vi "Display Lab Panel V9.vi"() -> ()   [LabVIEW 2017]
uses:
  Global display 1.vi
  Global display 3.vi
  Global display 2.vi
panel:
  out "network error":bool
  in  "Tab Control 2":T1(tab)
  out "SIG LAB05-2":T2 {"PF" format="%.2f"; "AMPS" format="%.1f"}
  out "SIG LAB05-1":T2 {"PF" format="%.2f"; "AMPS" format="%.1f"}
  out "SIG LAB04-2":T2 {"PF" format="%.2f"; "AMPS" format="%.1f"}
  out "SIG LAB04-1":T2 {"PF" format="%.2f"; "AMPS" format="%.1f"}
  out "SIG LAB03-2":T2 {"PF" format="%.2f"; "AMPS" format="%.1f"}
  out "SIG LAB03-1":T2 {"PF" format="%.2f"; "AMPS" format="%.1f"}
  out "SIG LAB02-2":T2 {"PF" format="%.2f"; "AMPS" format="%.1f"}
  in  "RUN LAB01-1":bool
  in  "O/I  LAB05-1":bool
  in  "O/I  LAB05-2":bool
  in  "O/I  LAB04-1":bool
  in  "O/I  LAB04-2":bool
  in  "O/I  LAB02-1":bool
  in  "O/I  LAB02-2":bool
  in  "O/I  LAB01-2":bool
  in  "O/I  LAB01-1":bool
  in  "O/I  LAB03-1":bool
  in  "RUN LAB05-2":bool
  in  "RUN LAB05-1":bool
  in  "RUN LAB04-2":bool
  in  "RUN LAB04-1":bool
  in  "RUN LAB03-2":bool
  in  "RUN LAB03-1":bool
  in  "RUN LAB02-2":bool
  in  "RUN LAB02-1":bool
  in  "RUN LAB01-2":bool
  in  "SELECT LAB05-2":T3(radio)
  in  "SELECT LAB05-1":T3(radio)
  in  "SELECT LAB04-2":T3(radio)
  in  "SELECT LAB04-1":T3(radio)
  in  "SELECT LAB03-2":T3(radio)
  in  "SELECT LAB03-1":T3(radio)
  in  "SELECT LAB02-2":T3(radio)
  in  "SELECT LAB02-1":T3(radio)
  in  "SELECT LAB01-2":T3(radio)
  in  "SELECT LAB01-1":T3(radio)
  in  "O/I  LAB03-2":bool
  out "SIG LAB01-1":T2 {"PF" format="%.2f"; "AMPS" format="%.1f"}
  out "SIG LAB01-2":T2 {"PF" format="%.2f"; "AMPS" format="%.1f"}
  out "SIG LAB02-1":T2 {"PF" format="%.2f"; "AMPS" format="%.1f"}
  out "DISP LAB05-2":T4 {"MINS" format="%.2g"}
  out "DISP LAB05-1":T4 {"MINS" format="%.2g"}
  out "DISP LAB04-2":T4 {"MINS" format="%.2g"}
  out "DISP LAB04-1":T4 {"MINS" format="%.2g"}
  out "DISP LAB03-2":T4 {"MINS" format="%.2g"}
  out "DISP LAB03-1":T4 {"MINS" format="%.2g"}
  in  "SET LAB05-2":T5={"NAME"="", "DESCRIPTION"="", "CYCLES"=5.0, "T-RISE mins"=0.0, "T-RISE deg C"=0.0} {"CYCLES" min=5.0 step=1.0}
  in  "SET LAB05-1":T5={"NAME"="", "DESCRIPTION"="", "CYCLES"=5.0, "T-RISE mins"=0.0, "T-RISE deg C"=0.0} {"CYCLES" min=5.0 step=1.0}
  in  "SET LAB04-2":T5={"NAME"="", "DESCRIPTION"="", "CYCLES"=5.0, "T-RISE mins"=0.0, "T-RISE deg C"=0.0} {"CYCLES" min=5.0 step=1.0}
  in  "SET LAB04-1":T5={"NAME"="", "DESCRIPTION"="", "CYCLES"=5.0, "T-RISE mins"=0.0, "T-RISE deg C"=0.0} {"CYCLES" min=5.0 step=1.0}
  in  "SET LAB03-2":T5={"NAME"="", "DESCRIPTION"="", "CYCLES"=5.0, "T-RISE mins"=0.0, "T-RISE deg C"=0.0} {"CYCLES" min=5.0 step=1.0}
  in  "SET LAB03-1":T5={"NAME"="", "DESCRIPTION"="", "CYCLES"=5.0, "T-RISE mins"=0.0, "T-RISE deg C"=0.0} {"CYCLES" min=5.0 step=1.0}
  out "DISP LAB02-2":T4 {"MINS" format="%.2g"}
  out "DISP LAB02-1":T4 {"MINS" format="%.2g"}
  in  "SET LAB02-2":T5={"NAME"="", "DESCRIPTION"="", "CYCLES"=5.0, "T-RISE mins"=0.0, "T-RISE deg C"=0.0} {"CYCLES" min=5.0 step=1.0}
  in  "SET LAB02-1":T5={"NAME"="", "DESCRIPTION"="", "CYCLES"=5.0, "T-RISE mins"=0.0, "T-RISE deg C"=0.0} {"CYCLES" min=5.0 step=1.0}
  out "RESULT LAB05-2":bool
  out "RESULT LAB05-1":bool
  out "RESULT LAB04-2":bool
  out "RESULT LAB04-1":bool
  out "RESULT LAB03-2":bool
  out "RESULT LAB03-1":bool
  out "RESULT LAB02-2":bool
  out "RESULT LAB02-1":bool
  out "RESULT LAB01-2":bool
  out "RESULT LAB01-1":bool
  in  "SET LAB01-1":T5={"NAME"="", "DESCRIPTION"="", "CYCLES"=5.0, "T-RISE mins"=0.0, "T-RISE deg C"=0.0} {"CYCLES" min=5.0 step=1.0}
  in  "SET LAB01-2":T5={"NAME"="", "DESCRIPTION"="", "CYCLES"=5.0, "T-RISE mins"=0.0, "T-RISE deg C"=0.0} {"CYCLES" min=5.0 step=1.0}
  out "DISP LAB01-1":T4 {"MINS" format="%.2g"}
  out "DISP LAB01-2":T4 {"MINS" format="%.2f"}
  out "TEMP RISE LAB05-2":cluster{"TL":dbl, "TN":dbl}
  out "TEMP RISE LAB05-1":cluster{"TL":dbl, "TN":dbl}
  out "TEMP RISE LAB04-2":cluster{"TL":dbl, "TN":dbl}
  out "TEMP RISE LAB04-1":cluster{"TL":dbl, "TN":dbl}
  out "TEMP RISE LAB03-2":cluster{"TL":dbl, "TN":dbl}
  out "TEMP RISE LAB03-1":cluster{"TL":dbl, "TN":dbl}
  out "TEMP RISE LAB02-2":cluster{"TL":dbl, "TN":dbl}
  out "TEMP RISE LAB02-1":cluster{"TL":dbl, "TN":dbl}
  out "TEMP RISE LAB01-2":cluster{"TL":dbl, "TN":dbl}
  out "TEMP RISE LAB01-1":cluster{"TL":dbl, "TN":dbl}
  out "TEMP START LAB01-1":cluster{"TL":dbl, "TN":dbl}
  out "TEMP START LAB02-1":cluster{"TL":dbl, "TN":dbl}
  out "TEMP START LAB03-1":cluster{"TL":dbl, "TN":dbl}
  out "TEMP START LAB04-1":cluster{"TL":dbl, "TN":dbl}
  out "TEMP START LAB01-2":cluster{"TL":dbl, "TN":dbl}
  out "TEMP START LAB02-2":cluster{"TL":dbl, "TN":dbl}
  out "TEMP START LAB03-2":cluster{"TL":dbl, "TN":dbl}
  out "TEMP START LAB04-2":cluster{"TL":dbl, "TN":dbl}
  out "TEMP START LAB05-2":cluster{"TL":dbl, "TN":dbl}
  out "TEMP START LAB05-1":cluster{"TL":dbl, "TN":dbl}
  in  "Save Log File\nTo Disk For\nViewing":bool
  out "LOG LAB05-2":string
  out "LOG LAB04-2":string
  out "LOG LAB03-2":string
  out "LOG LAB02-2":string
  out "LOG LAB01-2":string
  out "LOG LAB05-1":string
  out "LOG LAB04-1":string
  out "LOG LAB03-1":string
  out "LOG LAB02-1":string
  out "LOG LAB01-1":string
  out "LAB01 TEMP":dynamicdata(graph)
  out "LAB01 VOLTS":dynamicdata(graph)
  out "LAB01 AMPS":dynamicdata(graph)
  out "LAB02 TEMP":dynamicdata(graph)
  out "LAB02 VOLTS":dynamicdata(graph)
  out "LAB02 AMPS":dynamicdata(graph)
  out "LAB03 TEMP":dynamicdata(graph)
  out "LAB03 VOLTS":dynamicdata(graph)
  out "LAB03 AMPS":dynamicdata(graph)
  out "LAB04 TEMP":dynamicdata(graph)
  out "LAB04 VOLTS":dynamicdata(graph)
  out "LAB04 AMPS":dynamicdata(graph)
  out "LAB05 TEMP":dynamicdata(graph)
  out "LAB05 VOLTS":dynamicdata(graph)
  out "LAB05 AMPS":dynamicdata(graph)
  in  "Stop Button":bool
  out "log file dir":string
  out "log5-2":dbl
  out "log4-2":dbl
  out "log3-2":dbl
  out "log2-2":dbl
  out "log1-2":dbl
  out "log5-1":dbl
  out "log4-1":dbl
  out "log3-1":dbl
  out "log2-1":dbl
  out "log1-1":dbl
  out "graph update":bool
  out "LF5-2":bool
  out "LF5-1":bool
  out "LF3-2":bool
  out "LF3-1":bool
  out "LF4-2":bool
  out "LF4-1":bool
  out "LF2-2":bool
  out "LF2-1":bool
  out "LF1-2":bool
  out "LF1-1":bool
  out "error out":errorcluster
  # "LAB01"
  # "LAB02"
  # "LAB05"
  # "LAB03"
  # "LAB04"
  # "LAB01"
  # "LAB02"
  # "LAB03"
  # "LAB04"
  # "LAB05"
  # "PANEL ID / DATE / TIME / NAME / DESCRIPTION / CYCLES / TEST TIME / STATUS"
  # "PANEL ID / DATE / TIME / NAME / DESCRIPTION / CYCLES / TEST TIME / STATUS"
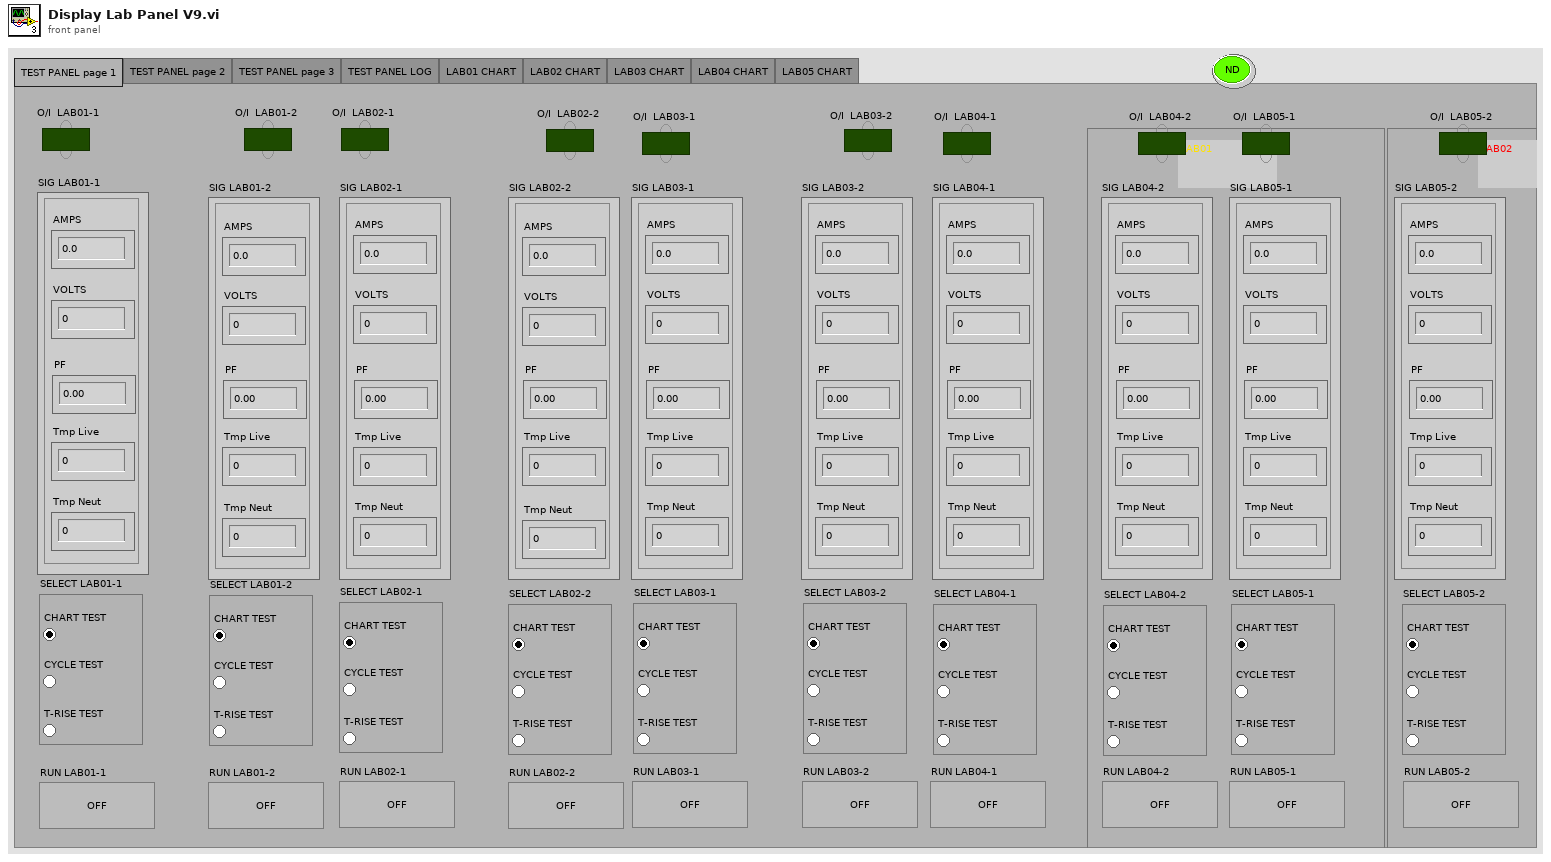
[diagram p1: front panel]
types:
  T1 = enum32{"TEST PANEL page 1", "TEST PANEL page 2", "TEST PANEL page 3", "TEST PANEL LOG", "LAB01 CHART", "LAB02 CHART", "LAB03 CHART", "LAB04 CHART", "LAB05 CHART", "ADM"}
  T2 = cluster{"AMPS":dbl, "VOLTS":dbl, "PF":dbl, "Tmp Live":dbl, "Tmp Neut":dbl}
  T3 = enum32{"CHART TEST", "CYCLE TEST", "T-RISE TEST"}
  T4 = cluster{"CYCLE":dbl, "MINS":dbl, "STATUS":string}
  T5 = cluster{"NAME":string, "DESCRIPTION":string, "CYCLES":dbl, "T-RISE mins":dbl, "T-RISE deg C":dbl}
  T6 = enum8{"Enabled", "Disabled", "Disabled and Grayed Out"}
  T7 = cluster{string, "date string":string, "time string":string, string, string, string, "STATUS":string}
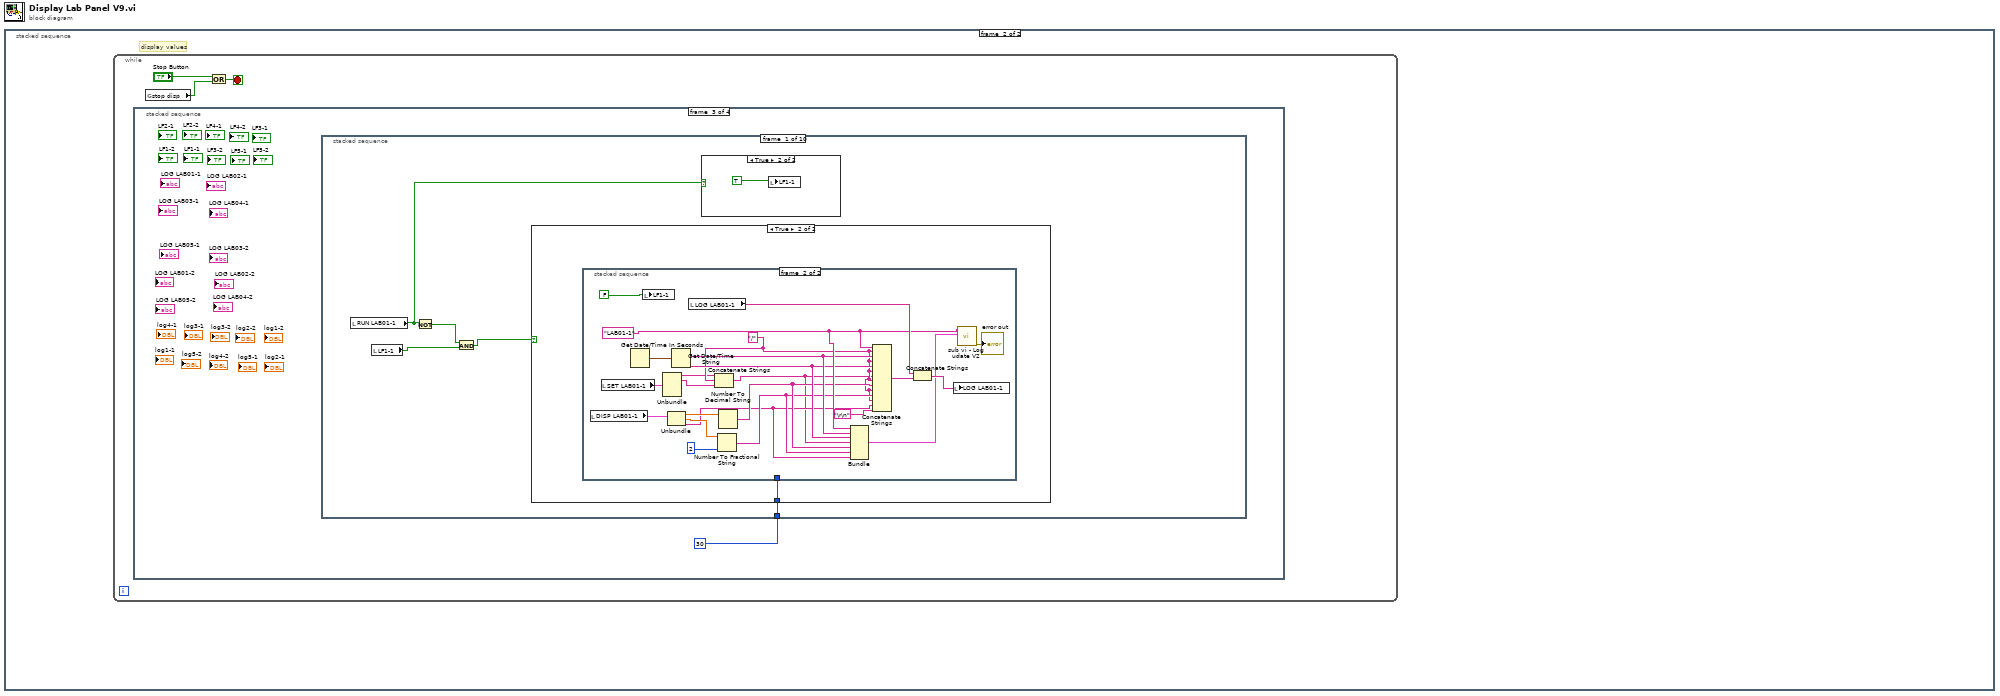
[diagram p0: block diagram]
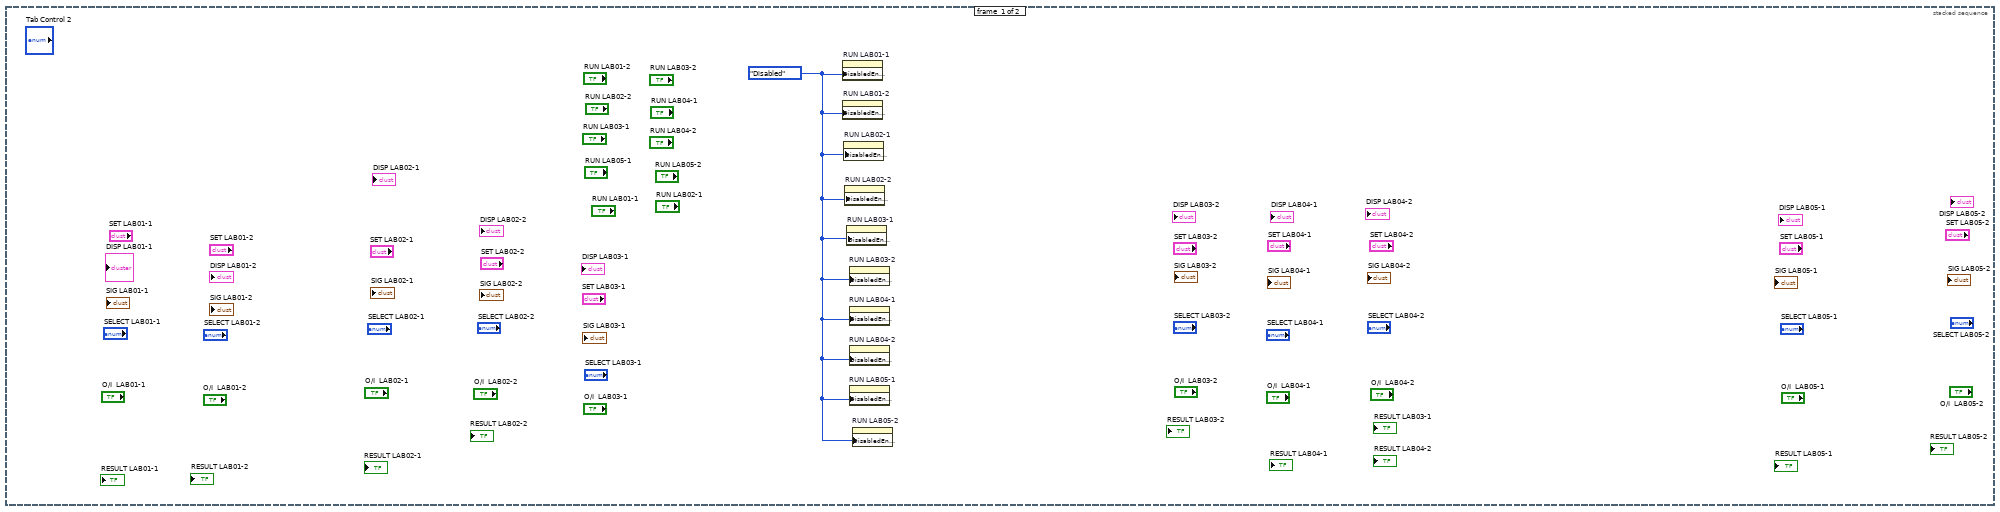
[diagram p2: hidden frame]
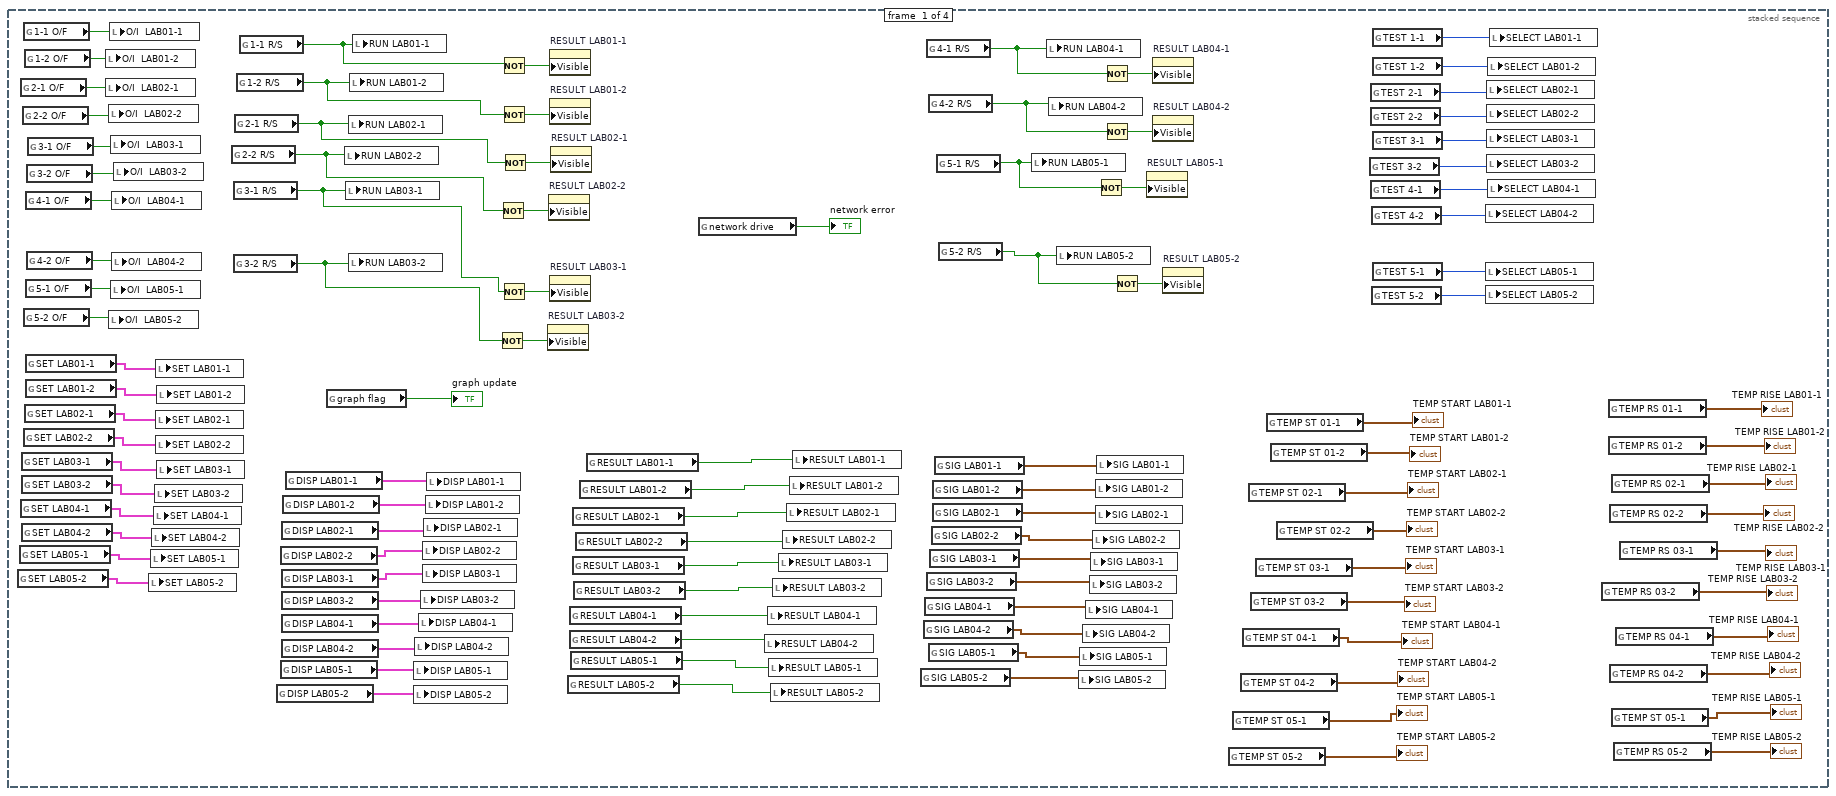
[diagram p3: hidden frame]
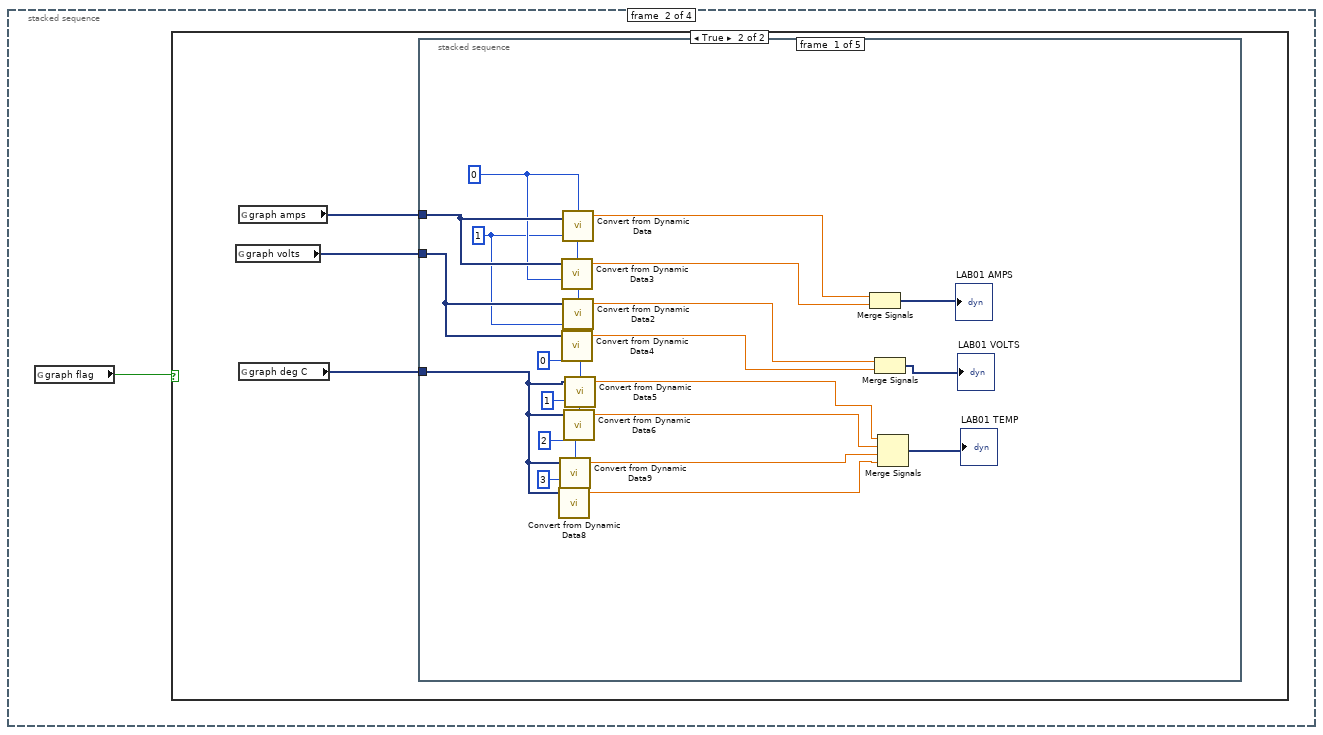
[diagram p4: hidden frame]
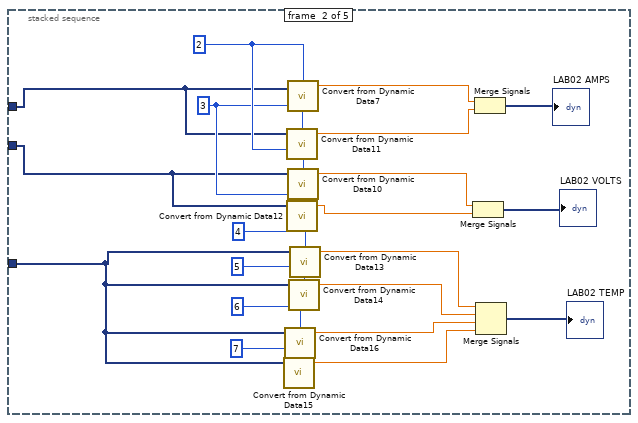
[diagram p6: hidden frame]
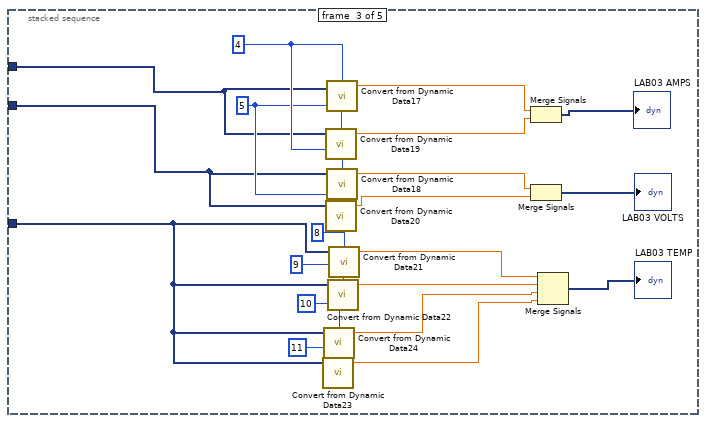
[diagram p7: hidden frame]
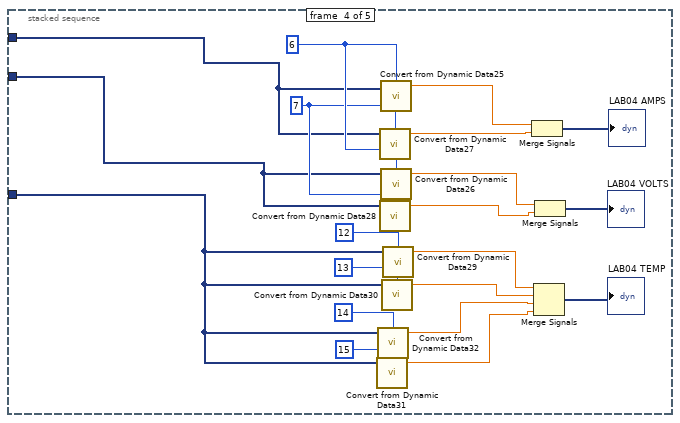
[diagram p8: hidden frame]
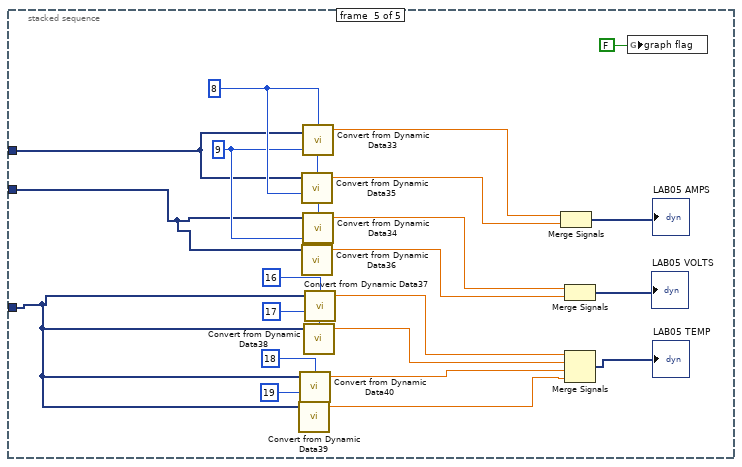
[diagram p9: hidden frame]
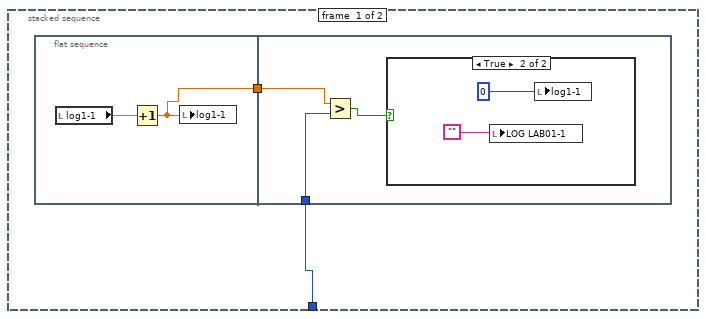
[diagram p11: hidden frame]
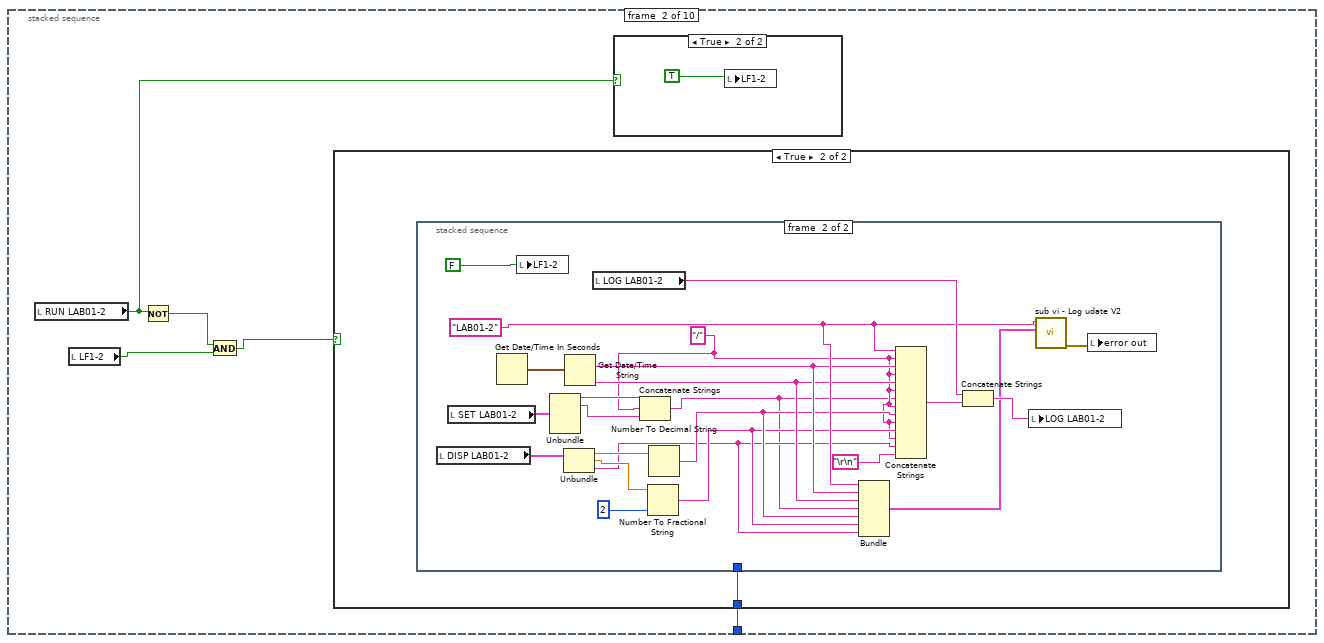
[diagram p14: hidden frame]
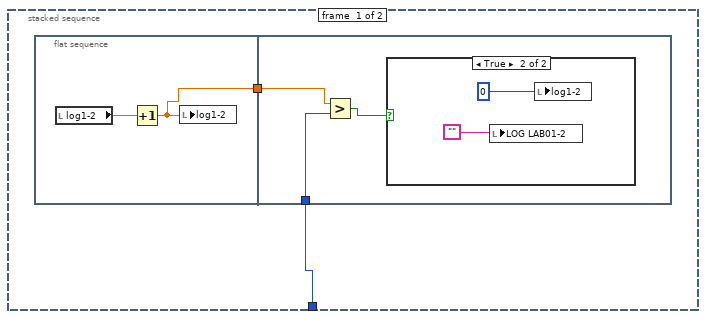
[diagram p16: hidden frame]
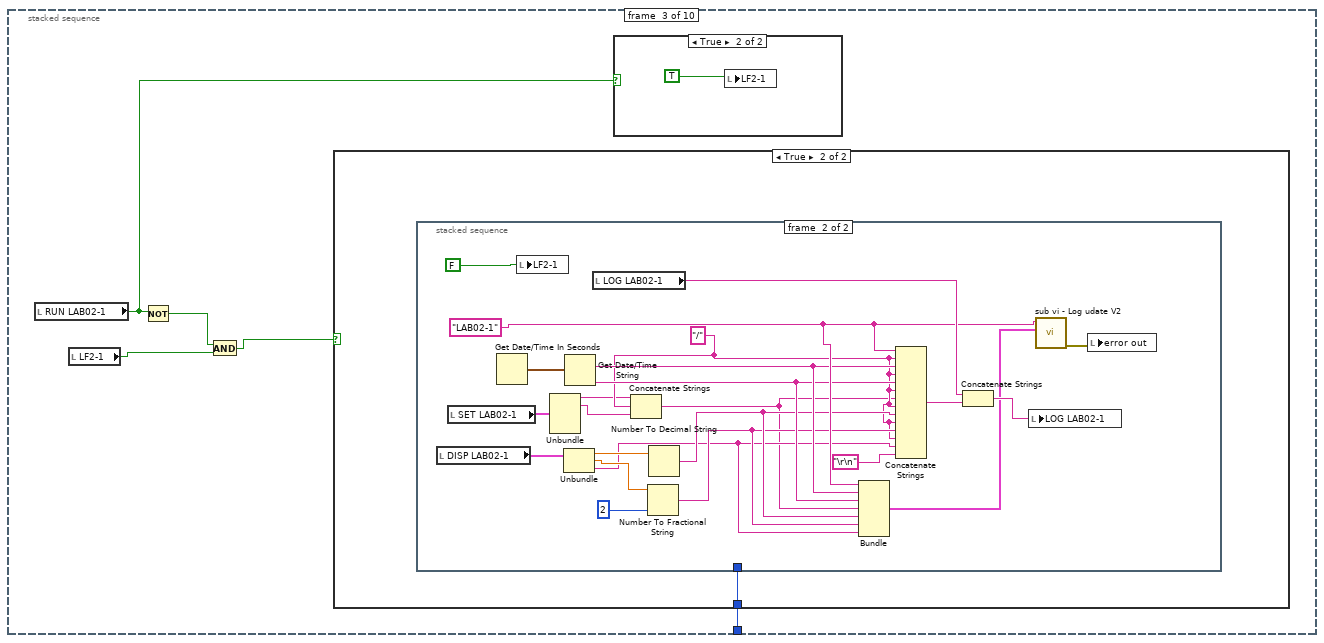
[diagram p19: hidden frame]
diagram:
  n1 = stacked-sequence {
    frame #0 {
      w1 = T6."Disabled" ("Disabled")
      n2 = property on="RUN LAB01-1" class="Bool (strict)"("DisabledEnum"=w1) -> ()  [unwired: 2 in, 2 out]
      n3 = property on="RUN LAB01-2" class="Bool (strict)"("DisabledEnum"=w1) -> ()  [unwired: 2 in, 2 out]
      n4 = property on="RUN LAB02-1" class="Bool (strict)"("DisabledEnum"=w1) -> ()  [unwired: 2 in, 2 out]
      n5 = property on="RUN LAB02-2" class="Bool (strict)"("DisabledEnum"=w1) -> ()  [unwired: 2 in, 2 out]
      n6 = property on="RUN LAB03-1" class="Bool (strict)"("DisabledEnum"=w1) -> ()  [unwired: 2 in, 2 out]
      n7 = property on="RUN LAB03-2" class="Bool (strict)"("DisabledEnum"=w1) -> ()  [unwired: 2 in, 2 out]
      n8 = property on="RUN LAB04-1" class="Bool (strict)"("DisabledEnum"=w1) -> ()  [unwired: 2 in, 2 out]
      n9 = property on="RUN LAB04-2" class="Bool (strict)"("DisabledEnum"=w1) -> ()  [unwired: 2 in, 2 out]
      n10 = property on="RUN LAB05-1" class="Bool (strict)"("DisabledEnum"=w1) -> ()  [unwired: 2 in, 2 out]
      n11 = property on="RUN LAB05-2" class="Bool (strict)"("DisabledEnum"=w1) -> ()  [unwired: 2 in, 2 out]
    }
    frame #1 {
      # "display values"
      n12 = while {
        stop <- w4 stop-if-true
        n13 = stacked-sequence {
          frame #0 {
            n14 = global read "Global display 2.vi" "SET LAB05-2"() -> (w67:T5)
            n15 = global read "Global display 2.vi" "SET LAB05-1"() -> (w68:T5)
            n16 = global read "Global display 1.vi" "2-1 O/F"() -> (w104:bool)
            n17 = global read "Global display 2.vi" "SET LAB04-1"() -> (w70:T5)
            n18 = global read "Global display 2.vi" "SET LAB03-1"() -> (w72:T5)
            n19 = global read "Global display 2.vi" "SET LAB03-2"() -> (w71:T5)
            n20 = global read "Global display 2.vi" "SET LAB04-2"() -> (w69:T5)
            n21 = global read "Global display 1.vi" "2-2 O/F"() -> (w103:bool)
            n22 = global read "Global display 1.vi" "1-1 O/F"() -> (w106:bool)
            n23 = global read "Global display 1.vi" "5-2 O/F"() -> (w97:bool)
            n24 = global read "Global display 2.vi" "SET LAB02-2"() -> (w73:T5)
            n25 = global read "Global display 1.vi" "1-2 O/F"() -> (w105:bool)
            n26 = global read "Global display 2.vi" "SET LAB02-1"() -> (w74:T5)
            n27 = global read "Global display 1.vi" "4-1 O/F"() -> (w100:bool)
            n28 = global read "Global display 1.vi" "5-1 O/F"() -> (w98:bool)
            n29 = global read "Global display 2.vi" "SET LAB01-1"() -> (w76:T5)
            n30 = global read "Global display 2.vi" "SET LAB01-2"() -> (w75:T5)
            n31 = global read "Global display 1.vi" "3-2 O/F"() -> (w101:bool)
            n32 = global read "Global display 1.vi" "4-2 O/F"() -> (w99:bool)
            n33 = global read "Global display 1.vi" "3-1 O/F"() -> (w102:bool)
            n34 = local write "O/I  LAB01-2"(w105) -> ()
            n35 = local write "O/I  LAB02-1"(w104) -> ()
            n36 = local write "O/I  LAB02-2"(w103) -> ()
            n37 = local write "O/I  LAB05-2"(w97) -> ()
            n38 = local write "O/I  LAB01-1"(w106) -> ()
            n39 = local write "O/I  LAB03-1"(w102) -> ()
            n40 = local write "O/I  LAB05-1"(w98) -> ()
            n41 = local write "O/I  LAB04-1"(w100) -> ()
            n42 = local write "O/I  LAB04-2"(w99) -> ()
            n43 = local write "O/I  LAB03-2"(w101) -> ()
            n44 = local write "SET LAB05-2"(w67) -> ()
            n45 = local write "SET LAB05-1"(w68) -> ()
            n46 = local write "SET LAB04-2"(w69) -> ()
            n47 = local write "SET LAB04-1"(w70) -> ()
            n48 = local write "SET LAB03-2"(w71) -> ()
            n49 = local write "SET LAB01-1"(w76) -> ()
            n50 = local write "SET LAB02-1"(w74) -> ()
            n51 = local write "SET LAB02-2"(w73) -> ()
            n52 = local write "SET LAB01-2"(w75) -> ()
            n53 = local write "SET LAB03-1"(w72) -> ()
            n54 = global read "Global display 1.vi" "2-2 R/S"() -> (w37:bool)
            n55 = global read "Global display 1.vi" "3-1 R/S"() -> (w36:bool)
            n56 = global read "Global display 1.vi" "3-2 R/S"() -> (w35:bool)
            n57 = global read "Global display 1.vi" "2-1 R/S"() -> (w38:bool)
            n58 = global read "Global display 1.vi" "1-2 R/S"() -> (w39:bool)
            n59 = global read "Global display 1.vi" "1-1 R/S"() -> (w45:bool)
            n60 = global read "Global display 2.vi" "DISP LAB05-2"() -> (w57:T4)
            n61 = global read "Global display 2.vi" "DISP LAB02-2"() -> (w63:T4)
            n62 = global read "Global display 2.vi" "DISP LAB05-1"() -> (w58:T4)
            n63 = global read "Global display 2.vi" "DISP LAB02-1"() -> (w64:T4)
            n64 = global read "Global display 2.vi" "DISP LAB03-1"() -> (w62:T4)
            n65 = global read "Global display 2.vi" "DISP LAB03-2"() -> (w61:T4)
            n66 = global read "Global display 2.vi" "DISP LAB04-1"() -> (w60:T4)
            n67 = global read "Global display 2.vi" "DISP LAB04-2"() -> (w59:T4)
            n68 = global read "Global display 2.vi" "DISP LAB01-2"() -> (w65:T4)
            n69 = global read "Global display 2.vi" "DISP LAB01-1"() -> (w66:T4)
            n70 = global read "Global display 3.vi" "graph flag"() -> (→"graph update":bool)
            n71 = local write "RUN LAB02-2"(w37) -> ()
            n72 = local write "RUN LAB03-1"(w36) -> ()
            n73 = local write "RUN LAB02-1"(w38) -> ()
            n74 = local write "RUN LAB03-2"(w35) -> ()
            n75 = local write "RUN LAB01-2"(w39) -> ()
            n76 = local write "RUN LAB01-1"(w45) -> ()
            n77 = local write "DISP LAB05-1"(w58) -> ()
            n78 = local write "DISP LAB05-2"(w57) -> ()
            n79 = local write "DISP LAB04-2"(w59) -> ()
            n80 = local write "DISP LAB04-1"(w60) -> ()
            n81 = local write "DISP LAB03-2"(w61) -> ()
            n82 = local write "DISP LAB02-2"(w63) -> ()
            n83 = local write "DISP LAB03-1"(w62) -> ()
            n84 = local write "DISP LAB02-1"(w64) -> ()
            n85 = local write "DISP LAB01-2"(w65) -> ()
            n86 = local write "DISP LAB01-1"(w66) -> ()
            n87 = Not(x=w35) -> (.not. x?=w40:bool)
            n88 = Not(x=w37) -> (.not. x?=w42:bool)
            n89 = Not(x=w45) -> (.not. x?=w46:bool)
            n90 = Not(x=w39) -> (.not. x?=w44:bool)
            n91 = Not(x=w36) -> (.not. x?=w41:bool)
            n92 = Not(x=w38) -> (.not. x?=w43:bool)
            n93 = property on="RESULT LAB03-2" class="Bool (strict)"("Visible"=w40) -> ()  [unwired: 2 in, 2 out]
            n94 = property on="RESULT LAB02-2" class="Bool (strict)"("Visible"=w42) -> ()  [unwired: 2 in, 2 out]
            n95 = property on="RESULT LAB01-1" class="Bool (strict)"("Visible"=w46) -> ()  [unwired: 2 in, 2 out]
            n96 = property on="RESULT LAB01-2" class="Bool (strict)"("Visible"=w44) -> ()  [unwired: 2 in, 2 out]
            n97 = property on="RESULT LAB03-1" class="Bool (strict)"("Visible"=w41) -> ()  [unwired: 2 in, 2 out]
            n98 = property on="RESULT LAB02-1" class="Bool (strict)"("Visible"=w43) -> ()  [unwired: 2 in, 2 out]
            n99 = global read "Global display 2.vi" "RESULT LAB05-2"() -> (w47:bool)
            n100 = global read "Global display 2.vi" "RESULT LAB04-1"() -> (w50:bool)
            n101 = global read "Global display 2.vi" "RESULT LAB04-2"() -> (w49:bool)
            n102 = global read "Global display 2.vi" "RESULT LAB05-1"() -> (w48:bool)
            n103 = global read "Global display 2.vi" "RESULT LAB02-1"() -> (w54:bool)
            n104 = global read "Global display 2.vi" "RESULT LAB03-1"() -> (w52:bool)
            n105 = global read "Global display 2.vi" "RESULT LAB03-2"() -> (w51:bool)
            n106 = global read "Global display 2.vi" "RESULT LAB02-2"() -> (w53:bool)
            n107 = global read "Global display 2.vi" "RESULT LAB01-2"() -> (w55:bool)
            n108 = global read "Global display 2.vi" "RESULT LAB01-1"() -> (w56:bool)
            n109 = global read "Global display 3.vi" "network drive"() -> (→"network error":bool)
            n110 = local write "RESULT LAB04-2"(w49) -> ()
            n111 = local write "RESULT LAB04-1"(w50) -> ()
            n112 = local write "RESULT LAB05-1"(w48) -> ()
            n113 = local write "RESULT LAB05-2"(w47) -> ()
            n114 = local write "RESULT LAB03-2"(w51) -> ()
            n115 = local write "RESULT LAB03-1"(w52) -> ()
            n116 = local write "RESULT LAB02-2"(w53) -> ()
            n117 = local write "RESULT LAB02-1"(w54) -> ()
            n118 = local write "RESULT LAB01-2"(w55) -> ()
            n119 = local write "RESULT LAB01-1"(w56) -> ()
            n120 = global read "Global display 1.vi" "SIG LAB05-2"() -> (w77:T2)
            n121 = global read "Global display 1.vi" "SIG LAB04-2"() -> (w79:T2)
            n122 = global read "Global display 1.vi" "SIG LAB04-1"() -> (w80:T2)
            n123 = global read "Global display 1.vi" "4-1 R/S"() -> (w33:bool)
            n124 = global read "Global display 1.vi" "SIG LAB03-2"() -> (w81:T2)
            n125 = global read "Global display 1.vi" "4-2 R/S"() -> (w31:bool)
            n126 = global read "Global display 1.vi" "SIG LAB05-1"() -> (w78:T2)
            n127 = global read "Global display 1.vi" "SIG LAB03-1"() -> (w82:T2)
            n128 = global read "Global display 1.vi" "SIG LAB02-2"() -> (w83:T2)
            n129 = global read "Global display 1.vi" "SIG LAB01-2"() -> (w85:T2)
            n130 = global read "Global display 1.vi" "SIG LAB02-1"() -> (w84:T2)
            n131 = global read "Global display 1.vi" "SIG LAB01-1"() -> (w86:T2)
            n132 = global read "Global display 1.vi" "5-1 R/S"() -> (w29:bool)
            n133 = global read "Global display 1.vi" "5-2 R/S"() -> (w27:bool)
            n134 = local write "RUN LAB05-1"(w29) -> ()
            n135 = local write "RUN LAB04-1"(w33) -> ()
            n136 = local write "RUN LAB04-2"(w31) -> ()
            n137 = local write "RUN LAB05-2"(w27) -> ()
            n138 = local write "SIG LAB05-2"(w77) -> ()
            n139 = local write "SIG LAB05-1"(w78) -> ()
            n140 = local write "SIG LAB04-2"(w79) -> ()
            n141 = local write "SIG LAB04-1"(w80) -> ()
            n142 = local write "SIG LAB03-2"(w81) -> ()
            n143 = local write "SIG LAB03-1"(w82) -> ()
            n144 = local write "SIG LAB02-2"(w83) -> ()
            n145 = Not(x=w29) -> (.not. x?=w30:bool)
            n146 = local write "SIG LAB01-2"(w85) -> ()
            n147 = local write "SIG LAB02-1"(w84) -> ()
            n148 = local write "SIG LAB01-1"(w86) -> ()
            n149 = Not(x=w33) -> (.not. x?=w34:bool)
            n150 = Not(x=w31) -> (.not. x?=w32:bool)
            n151 = Not(x=w27) -> (.not. x?=w28:bool)
            n152 = property on="RESULT LAB05-1" class="Bool (strict)"("Visible"=w30) -> ()  [unwired: 2 in, 2 out]
            n153 = property on="RESULT LAB04-1" class="Bool (strict)"("Visible"=w34) -> ()  [unwired: 2 in, 2 out]
            n154 = property on="RESULT LAB04-2" class="Bool (strict)"("Visible"=w32) -> ()  [unwired: 2 in, 2 out]
            n155 = property on="RESULT LAB05-2" class="Bool (strict)"("Visible"=w28) -> ()  [unwired: 2 in, 2 out]
            n156 = global read "Global display 3.vi" "TEMP ST 05-2"() -> (→"TEMP START LAB05-2":cluster{"TL":dbl, "TN":dbl})
            n157 = global read "Global display 3.vi" "TEMP ST 05-1"() -> (→"TEMP START LAB05-1":cluster{"TL":dbl, "TN":dbl})
            n158 = global read "Global display 3.vi" "TEMP ST 04-2"() -> (→"TEMP START LAB04-2":cluster{"TL":dbl, "TN":dbl})
            n159 = global read "Global display 3.vi" "TEMP ST 04-1"() -> (→"TEMP START LAB04-1":cluster{"TL":dbl, "TN":dbl})
            n160 = global read "Global display 3.vi" "TEMP ST 02-1"() -> (→"TEMP START LAB02-1":cluster{"TL":dbl, "TN":dbl})
            n161 = global read "Global display 3.vi" "TEMP ST 03-2"() -> (→"TEMP START LAB03-2":cluster{"TL":dbl, "TN":dbl})
            n162 = global read "Global display 3.vi" "TEMP ST 03-1"() -> (→"TEMP START LAB03-1":cluster{"TL":dbl, "TN":dbl})
            n163 = global read "Global display 3.vi" "TEMP ST 01-1"() -> (→"TEMP START LAB01-1":cluster{"TL":dbl, "TN":dbl})
            n164 = global read "Global display 3.vi" "TEMP ST 01-2"() -> (→"TEMP START LAB01-2":cluster{"TL":dbl, "TN":dbl})
            n165 = global read "Global display 3.vi" "TEMP ST 02-2"() -> (→"TEMP START LAB02-2":cluster{"TL":dbl, "TN":dbl})
            n166 = global read "Global display 1.vi" "TEST 3-2"() -> (w91:T3)
            n167 = global read "Global display 1.vi" "TEST 2-1"() -> (w94:T3)
            n168 = global read "Global display 1.vi" "TEST 2-2"() -> (w93:T3)
            n169 = global read "Global display 1.vi" "TEST 4-1"() -> (w90:T3)
            n170 = global read "Global display 1.vi" "TEST 4-2"() -> (w89:T3)
            n171 = global read "Global display 1.vi" "TEST 5-2"() -> (w87:T3)
            n172 = global read "Global display 1.vi" "TEST 1-1"() -> (w96:T3)
            n173 = global read "Global display 1.vi" "TEST 1-2"() -> (w95:T3)
            n174 = global read "Global display 1.vi" "TEST 3-1"() -> (w92:T3)
            n175 = global read "Global display 1.vi" "TEST 5-1"() -> (w88:T3)
            n176 = local write "SELECT LAB04-2"(w89) -> ()
            n177 = local write "SELECT LAB05-1"(w88) -> ()
            n178 = local write "SELECT LAB05-2"(w87) -> ()
            n179 = local write "SELECT LAB02-1"(w94) -> ()
            n180 = local write "SELECT LAB02-2"(w93) -> ()
            n181 = local write "SELECT LAB03-1"(w92) -> ()
            n182 = local write "SELECT LAB03-2"(w91) -> ()
            n183 = local write "SELECT LAB01-2"(w95) -> ()
            n184 = local write "SELECT LAB04-1"(w90) -> ()
            n185 = local write "SELECT LAB01-1"(w96) -> ()
            n186 = global read "Global display 3.vi" "TEMP RS 03-2"() -> (→"TEMP RISE LAB03-2":cluster{"TL":dbl, "TN":dbl})
            n187 = global read "Global display 3.vi" "TEMP RS 01-1"() -> (→"TEMP RISE LAB01-1":cluster{"TL":dbl, "TN":dbl})
            n188 = global read "Global display 3.vi" "TEMP RS 01-2"() -> (→"TEMP RISE LAB01-2":cluster{"TL":dbl, "TN":dbl})
            n189 = global read "Global display 3.vi" "TEMP RS 02-2"() -> (→"TEMP RISE LAB02-2":cluster{"TL":dbl, "TN":dbl})
            n190 = global read "Global display 3.vi" "TEMP RS 04-2"() -> (→"TEMP RISE LAB04-2":cluster{"TL":dbl, "TN":dbl})
            n191 = global read "Global display 3.vi" "TEMP RS 02-1"() -> (→"TEMP RISE LAB02-1":cluster{"TL":dbl, "TN":dbl})
            n192 = global read "Global display 3.vi" "TEMP ST 05-1"() -> (→"TEMP RISE LAB05-1":cluster{"TL":dbl, "TN":dbl})
            n193 = global read "Global display 3.vi" "TEMP RS 05-2"() -> (→"TEMP RISE LAB05-2":cluster{"TL":dbl, "TN":dbl})
            n194 = global read "Global display 3.vi" "TEMP RS 04-1"() -> (→"TEMP RISE LAB04-1":cluster{"TL":dbl, "TN":dbl})
            n195 = global read "Global display 3.vi" "TEMP RS 03-1"() -> (→"TEMP RISE LAB03-1":cluster{"TL":dbl, "TN":dbl})
          }
          frame #1 {
            n196 = global read "Global display 3.vi" "graph flag"() -> (w107:bool)
            n197 = case shown="True" w107 {
              frame False {
              }
              frame True {
                n198 = global read "Global display 3.vi" "graph volts"() -> (w109:dynamicdata)
                n199 = global read "Global display 3.vi" "graph amps"() -> (w110:dynamicdata)
                n200 = global read "Global display 3.vi" "graph deg C"() -> (w108:dynamicdata)
                n201 = stacked-sequence {
                  tunnel: w110 -> [w127 w145 w165 w185 w205]
                  tunnel: w109 -> [w124 w144 w164 w184 w204]
                  tunnel: w108 -> [w119 w139 w155 w179 w195]
                  frame #0 {
                    w120 = 1
                    w121 = 0
                    n202 = call "Convert from Dynamic Data8"("Dynamic Data Type"=w119, "Channel"=3) -> ("Scalar"=w111:dbl)  [unwired: 2 in]
                    n203 = call "Convert from Dynamic Data9"("Dynamic Data Type"=w119, "Channel"=2) -> ("Scalar"=w112:dbl)  [unwired: 2 in]
                    n204 = call "Convert from Dynamic Data3"("Dynamic Data Type"=w127, "Channel"=w120) -> ("Scalar"=w125:dbl)  [unwired: 2 in]
                    n205 = call "Convert from Dynamic Data4"("Dynamic Data Type"=w124, "Channel"=w120) -> ("Scalar"=w122:dbl)  [unwired: 2 in]
                    n206 = call "Convert from Dynamic Data"("Dynamic Data Type"=w127, "Channel"=w121) -> ("Scalar"=w126:dbl)  [unwired: 2 in]
                    n207 = call "Convert from Dynamic Data2"("Dynamic Data Type"=w124, "Channel"=w121) -> ("Scalar"=w123:dbl)  [unwired: 2 in]
                    n208 = call "Convert from Dynamic Data6"("Dynamic Data Type"=w119, "Channel"=1) -> ("Scalar"=w113:dbl)  [unwired: 2 in]
                    n209 = call "Convert from Dynamic Data5"("Dynamic Data Type"=w119, "Channel"=0) -> ("Scalar"=w114:dbl)  [unwired: 2 in]
                    n210 = Merge Signals(w126, w125) -> (→"LAB01 AMPS":dynamicdata)
                    n211 = Merge Signals(w123, w122) -> (→"LAB01 VOLTS":dynamicdata)
                    n212 = Merge Signals(w114, w113, w112, w111) -> (→"LAB01 TEMP":dynamicdata)
                  }
                  frame #1 {
                    w149 = 3
                    w150 = 2
                    n213 = call "Convert from Dynamic Data15"("Dynamic Data Type"=w139, "Channel"=7) -> ("Scalar"=w135:dbl)  [unwired: 2 in]
                    n214 = call "Convert from Dynamic Data16"("Dynamic Data Type"=w139, "Channel"=6) -> ("Scalar"=w136:dbl)  [unwired: 2 in]
                    n215 = call "Convert from Dynamic Data11"("Dynamic Data Type"=w145, "Channel"=w149) -> ("Scalar"=w142:dbl)  [unwired: 2 in]
                    n216 = call "Convert from Dynamic Data12"("Dynamic Data Type"=w144, "Channel"=w149) -> ("Scalar"=w140:dbl)  [unwired: 2 in]
                    n217 = call "Convert from Dynamic Data7"("Dynamic Data Type"=w145, "Channel"=w150) -> ("Scalar"=w143:dbl)  [unwired: 2 in]
                    n218 = call "Convert from Dynamic Data10"("Dynamic Data Type"=w144, "Channel"=w150) -> ("Scalar"=w141:dbl)  [unwired: 2 in]
                    n219 = call "Convert from Dynamic Data14"("Dynamic Data Type"=w139, "Channel"=5) -> ("Scalar"=w137:dbl)  [unwired: 2 in]
                    n220 = call "Convert from Dynamic Data13"("Dynamic Data Type"=w139, "Channel"=4) -> ("Scalar"=w138:dbl)  [unwired: 2 in]
                    n221 = Merge Signals(w141, w140) -> (→"LAB02 VOLTS":dynamicdata)
                    n222 = Merge Signals(w143, w142) -> (→"LAB02 AMPS":dynamicdata)
                    n223 = Merge Signals(w138, w137, w136, w135) -> (→"LAB02 TEMP":dynamicdata)
                  }
                  frame #2 {
                    w169 = 5
                    w170 = 4
                    n224 = call "Convert from Dynamic Data23"("Dynamic Data Type"=w155, "Channel"=11) -> ("Scalar"=w156:dbl)  [unwired: 2 in]
                    n225 = call "Convert from Dynamic Data24"("Dynamic Data Type"=w155, "Channel"=10) -> ("Scalar"=w157:dbl)  [unwired: 2 in]
                    n226 = call "Convert from Dynamic Data19"("Dynamic Data Type"=w165, "Channel"=w169) -> ("Scalar"=w162:dbl)  [unwired: 2 in]
                    n227 = call "Convert from Dynamic Data20"("Dynamic Data Type"=w164, "Channel"=w169) -> ("Scalar"=w160:dbl)  [unwired: 2 in]
                    n228 = call "Convert from Dynamic Data17"("Dynamic Data Type"=w165, "Channel"=w170) -> ("Scalar"=w163:dbl)  [unwired: 2 in]
                    n229 = call "Convert from Dynamic Data18"("Dynamic Data Type"=w164, "Channel"=w170) -> ("Scalar"=w161:dbl)  [unwired: 2 in]
                    n230 = call "Convert from Dynamic Data22"("Dynamic Data Type"=w155, "Channel"=9) -> ("Scalar"=w158:dbl)  [unwired: 2 in]
                    n231 = call "Convert from Dynamic Data21"("Dynamic Data Type"=w155, "Channel"=8) -> ("Scalar"=w159:dbl)  [unwired: 2 in]
                    n232 = Merge Signals(w163, w162) -> (→"LAB03 AMPS":dynamicdata)
                    n233 = Merge Signals(w161, w160) -> (→"LAB03 VOLTS":dynamicdata)
                    n234 = Merge Signals(w159, w158, w157, w156) -> (→"LAB03 TEMP":dynamicdata)
                  }
                  frame #3 {
                    w186 = 7
                    w187 = 6
                    n235 = call "Convert from Dynamic Data31"("Dynamic Data Type"=w179, "Channel"=15) -> ("Scalar"=w175:dbl)  [unwired: 2 in]
                    n236 = call "Convert from Dynamic Data32"("Dynamic Data Type"=w179, "Channel"=14) -> ("Scalar"=w176:dbl)  [unwired: 2 in]
                    n237 = call "Convert from Dynamic Data27"("Dynamic Data Type"=w185, "Channel"=w186) -> ("Scalar"=w182:dbl)  [unwired: 2 in]
                    n238 = call "Convert from Dynamic Data28"("Dynamic Data Type"=w184, "Channel"=w186) -> ("Scalar"=w180:dbl)  [unwired: 2 in]
                    n239 = call "Convert from Dynamic Data25"("Dynamic Data Type"=w185, "Channel"=w187) -> ("Scalar"=w183:dbl)  [unwired: 2 in]
                    n240 = call "Convert from Dynamic Data26"("Dynamic Data Type"=w184, "Channel"=w187) -> ("Scalar"=w181:dbl)  [unwired: 2 in]
                    n241 = call "Convert from Dynamic Data30"("Dynamic Data Type"=w179, "Channel"=13) -> ("Scalar"=w177:dbl)  [unwired: 2 in]
                    n242 = call "Convert from Dynamic Data29"("Dynamic Data Type"=w179, "Channel"=12) -> ("Scalar"=w178:dbl)  [unwired: 2 in]
                    n243 = Merge Signals(w183, w182) -> (→"LAB04 AMPS":dynamicdata)
                    n244 = Merge Signals(w178, w177, w176, w175) -> (→"LAB04 TEMP":dynamicdata)
                    n245 = Merge Signals(w181, w180) -> (→"LAB04 VOLTS":dynamicdata)
                  }
                  frame #4 {
                    w209 = 9
                    w210 = 8
                    n246 = call "Convert from Dynamic Data39"("Dynamic Data Type"=w195, "Channel"=19) -> ("Scalar"=w196:dbl)  [unwired: 2 in]
                    n247 = call "Convert from Dynamic Data40"("Dynamic Data Type"=w195, "Channel"=18) -> ("Scalar"=w197:dbl)  [unwired: 2 in]
                    n248 = call "Convert from Dynamic Data35"("Dynamic Data Type"=w205, "Channel"=w209) -> ("Scalar"=w202:dbl)  [unwired: 2 in]
                    n249 = call "Convert from Dynamic Data36"("Dynamic Data Type"=w204, "Channel"=w209) -> ("Scalar"=w200:dbl)  [unwired: 2 in]
                    n250 = call "Convert from Dynamic Data33"("Dynamic Data Type"=w205, "Channel"=w210) -> ("Scalar"=w203:dbl)  [unwired: 2 in]
                    n251 = call "Convert from Dynamic Data34"("Dynamic Data Type"=w204, "Channel"=w210) -> ("Scalar"=w201:dbl)  [unwired: 2 in]
                    n252 = call "Convert from Dynamic Data38"("Dynamic Data Type"=w195, "Channel"=17) -> ("Scalar"=w198:dbl)  [unwired: 2 in]
                    n253 = call "Convert from Dynamic Data37"("Dynamic Data Type"=w195, "Channel"=16) -> ("Scalar"=w199:dbl)  [unwired: 2 in]
                    n254 = Merge Signals(w203, w202) -> (→"LAB05 AMPS":dynamicdata)
                    n255 = Merge Signals(w201, w200) -> (→"LAB05 VOLTS":dynamicdata)
                    n256 = Merge Signals(w199, w198, w197, w196) -> (→"LAB05 TEMP":dynamicdata)
                    n257 = global write "Global display 3.vi" "graph flag"(FALSE) -> ()
                  }
                }
              }
            }
          }
          frame #2 {
            n258 = stacked-sequence {
              tunnel: 30 -> [w213 w252 w291 w330 w369 w408 w447 w486 w525 w564]
              frame #0 {
                n259 = local read "RUN LAB01-1"() -> (w214:bool)
                n260 = local read "LF1-1"() -> (w216:bool)
                n261 = Not(x=w214) -> (.not. x?=w217:bool)
                n262 = And(x=w217, y=w216) -> (x .and. y?=w215:bool)
                n263 = case shown="True" w215 {
                  tunnel: w213 -> [_ w218]
                  frame False {
                  }
                  frame True {
                    n264 = stacked-sequence {
                      tunnel: w218 -> [w219 _]
                      frame #0 {
                        n265 = flat-sequence {
                          tunnel: [w221] -> w220
                          tunnel: w220 -> [w224]
                          tunnel: w219 -> [w223]
                          frame #0 {
                            n266 = local read "log1-1"() -> (w222:dbl)
                            n267 = Increment(x=w222) -> (x+1=w221:dbl)
                            n268 = local write "log1-1"(w221) -> ()
                          }
                          frame #1 {
                            n269 = Greater?(x=w224, y=w223) -> (0:w225:bool)
                            n270 = case shown="True" w225 {
                              frame False {
                              }
                              frame True {
                                n271 = local write "LOG LAB01-1"("") -> ()
                                n272 = local write "log1-1"(0) -> ()
                              }
                            }
                          }
                        }
                      }
                      frame #1 {
                        w239 = "LAB01-1"
                        w231 = "/"
                        n273 = local read "DISP LAB01-1"() -> (w249:T4)
                        n274 = local read "SET LAB01-1"() -> (w243:T5)
                        n275 = Get Date/Time In Seconds() -> (seconds since 1Jan1904=w245:timestamp)
                        n276 = local write "LF1-1"(FALSE) -> ()
                        n277 = Unbundle(w243) -> ("NAME"=w230:string, "DESCRIPTION"=w229:string)  [unwired: 3 out]
                        n278 = Unbundle(w249) -> ("CYCLE"=w248:dbl, "MINS"=w247:dbl, "STATUS"=w234:string)
                        n279 = Get Date/Time String(seconds (now)=w245) -> (date string=w238:string, time string=w237:string)  [unwired: 2 in]
                        n280 = local read "LOG LAB01-1"() -> (w242:string)
                        n281 = Concatenate Strings(w230, w231, w229) -> (w228:string)
                        n282 = Number To Fractional String(number=w247, precision (6)=2) -> (F-format string=w235:string)  [unwired: 2 in]
                        n283 = Number To Decimal String(number=w248) -> (decimal integer string=w236:string)  [unwired: 1 in]
                        n284 = Bundle(w239, "date string"=w238, "time string"=w237, w228, w236, w235, "STATUS"=w234) -> (w233:T7)  [unwired: 1 in]
                        n285 = Concatenate Strings(w239, w231, w238, w231, w237, w231, w228, w231, w236, w231, w235, w231, w234, "\r\n") -> (w240:string)
                        n286 = Concatenate Strings(w242, w240) -> (w241:string)
                        n287 = local write "LOG LAB01-1"(w241) -> ()
                        n288 = call "sub vi - Log udate V2.vi"("data"=w233, "panel id"=w239) -> ("error out"=→"error out":errorcluster)  [unwired: 9 in]
                      }
                    }
                  }
                }
                n289 = case shown="True" w214 {
                  frame False {
                  }
                  frame True {
                    n290 = local write "LF1-1"(TRUE) -> ()
                  }
                }
              }
              frame #1 {
                n291 = local read "RUN LAB01-2"() -> (w253:bool)
                n292 = local read "LF1-2"() -> (w255:bool)
                n293 = Not(x=w253) -> (.not. x?=w256:bool)
                n294 = And(x=w256, y=w255) -> (x .and. y?=w254:bool)
                n295 = case shown="True" w254 {
                  tunnel: w252 -> [_ w257]
                  frame False {
                  }
                  frame True {
                    n296 = stacked-sequence {
                      tunnel: w257 -> [w258 _]
                      frame #0 {
                        n297 = flat-sequence {
                          tunnel: [w260] -> w259
                          tunnel: w259 -> [w263]
                          tunnel: w258 -> [w262]
                          frame #0 {
                            n298 = local read "log1-2"() -> (w261:dbl)
                            n299 = Increment(x=w261) -> (x+1=w260:dbl)
                            n300 = local write "log1-2"(w260) -> ()
                          }
                          frame #1 {
                            n301 = Greater?(x=w263, y=w262) -> (0:w264:bool)
                            n302 = case shown="True" w264 {
                              frame False {
                              }
                              frame True {
                                n303 = local write "LOG LAB01-2"("") -> ()
                                n304 = local write "log1-2"(0) -> ()
                              }
                            }
                          }
                        }
                      }
                      frame #1 {
                        w278 = "LAB01-2"
                        w269 = "/"
                        n305 = local read "DISP LAB01-2"() -> (w288:T4)
                        n306 = local read "SET LAB01-2"() -> (w282:T5)
                        n307 = Get Date/Time In Seconds() -> (seconds since 1Jan1904=w284:timestamp)
                        n308 = local write "LF1-2"(FALSE) -> ()
                        n309 = Unbundle(w282) -> ("NAME"=w270:string, "DESCRIPTION"=w268:string)  [unwired: 3 out]
                        n310 = Unbundle(w288) -> ("CYCLE"=w287:dbl, "MINS"=w286:dbl, "STATUS"=w273:string)
                        n311 = Get Date/Time String(seconds (now)=w284) -> (date string=w277:string, time string=w276:string)  [unwired: 2 in]
                        n312 = local read "LOG LAB01-2"() -> (w281:string)
                        n313 = Concatenate Strings(w270, w269, w268) -> (w267:string)
                        n314 = Number To Fractional String(number=w286, precision (6)=2) -> (F-format string=w274:string)  [unwired: 2 in]
                        n315 = Number To Decimal String(number=w287) -> (decimal integer string=w275:string)  [unwired: 1 in]
                        n316 = Bundle(w278, "date string"=w277, "time string"=w276, w267, w275, w274, "STATUS"=w273) -> (w272:T7)  [unwired: 1 in]
                        n317 = Concatenate Strings(w278, w269, w277, w269, w276, w269, w267, w269, w275, w269, w274, w269, w273, "\r\n") -> (w279:string)
                        n318 = Concatenate Strings(w281, w279) -> (w280:string)
                        n319 = local write "LOG LAB01-2"(w280) -> ()
                        n320 = call "sub vi - Log udate V2.vi"("data"=w272, "panel id"=w278) -> ("error out"=w271:errorcluster)  [unwired: 9 in]
                        n321 = local write "error out"(w271) -> ()
                      }
                    }
                  }
                }
                n322 = case shown="True" w253 {
                  frame False {
                  }
                  frame True {
                    n323 = local write "LF1-2"(TRUE) -> ()
                  }
                }
              }
              frame #2 {
                n324 = local read "RUN LAB02-1"() -> (w292:bool)
                n325 = local read "LF2-1"() -> (w294:bool)
                n326 = Not(x=w292) -> (.not. x?=w295:bool)
                n327 = And(x=w295, y=w294) -> (x .and. y?=w293:bool)
                n328 = case shown="True" w293 {
                  tunnel: w291 -> [_ w296]
                  frame False {
                  }
                  frame True {
                    n329 = stacked-sequence {
                      tunnel: w296 -> [w297 _]
                      frame #0 {
                        n330 = flat-sequence {
                          tunnel: [w299] -> w298
                          tunnel: w298 -> [w302]
                          tunnel: w297 -> [w301]
                          frame #0 {
                            n331 = local read "log2-1"() -> (w300:dbl)
                            n332 = Increment(x=w300) -> (x+1=w299:dbl)
                            n333 = local write "log2-1"(w299) -> ()
                          }
                          frame #1 {
                            n334 = Greater?(x=w302, y=w301) -> (0:w303:bool)
                            n335 = case shown="True" w303 {
                              frame False {
                              }
                              frame True {
                                n336 = local write "LOG LAB02-1"("") -> ()
                                n337 = local write "log2-1"(0) -> ()
                              }
                            }
                          }
                        }
                      }
                      frame #1 {
                        w317 = "LAB02-1"
                        w309 = "/"
                        n338 = local read "DISP LAB02-1"() -> (w327:T4)
                        n339 = local read "SET LAB02-1"() -> (w321:T5)
                        n340 = Get Date/Time In Seconds() -> (seconds since 1Jan1904=w323:timestamp)
                        n341 = local write "LF2-1"(FALSE) -> ()
                        n342 = Unbundle(w321) -> ("NAME"=w308:string, "DESCRIPTION"=w307:string)  [unwired: 3 out]
                        n343 = Unbundle(w327) -> ("CYCLE"=w326:dbl, "MINS"=w325:dbl, "STATUS"=w312:string)
                        n344 = Get Date/Time String(seconds (now)=w323) -> (date string=w316:string, time string=w315:string)  [unwired: 2 in]
                        n345 = local read "LOG LAB02-1"() -> (w320:string)
                        n346 = Concatenate Strings(w308, w309, w307) -> (w306:string)
                        n347 = Number To Fractional String(number=w325, precision (6)=2) -> (F-format string=w313:string)  [unwired: 2 in]
                        n348 = Number To Decimal String(number=w326) -> (decimal integer string=w314:string)  [unwired: 1 in]
                        n349 = Bundle(w317, "date string"=w316, "time string"=w315, w306, w314, w313, "STATUS"=w312) -> (w311:T7)  [unwired: 1 in]
                        n350 = Concatenate Strings(w317, w309, w316, w309, w315, w309, w306, w309, w314, w309, w313, w309, w312, "\r\n") -> (w318:string)
                        n351 = Concatenate Strings(w320, w318) -> (w319:string)
                        n352 = local write "LOG LAB02-1"(w319) -> ()
                        n353 = call "sub vi - Log udate V2.vi"("data"=w311, "panel id"=w317) -> ("error out"=w310:errorcluster)  [unwired: 9 in]
                        n354 = local write "error out"(w310) -> ()
                      }
                    }
                  }
                }
                n355 = case shown="True" w292 {
                  frame False {
                  }
                  frame True {
                    n356 = local write "LF2-1"(TRUE) -> ()
                  }
                }
              }
              frame #3 {
                n357 = local read "RUN LAB02-2"() -> (w331:bool)
                n358 = local read "LF2-2"() -> (w333:bool)
                n359 = Not(x=w331) -> (.not. x?=w334:bool)
                n360 = And(x=w334, y=w333) -> (x .and. y?=w332:bool)
                n361 = case shown="True" w332 {
                  tunnel: w330 -> [_ w335]
                  frame False {
                  }
                  frame True {
                    n362 = stacked-sequence {
                      tunnel: w335 -> [w336 _]
                      frame #0 {
                        n363 = flat-sequence {
                          tunnel: [w338] -> w337
                          tunnel: w337 -> [w341]
                          tunnel: w336 -> [w340]
                          frame #0 {
                            n364 = local read "log2-2"() -> (w339:dbl)
                            n365 = Increment(x=w339) -> (x+1=w338:dbl)
                            n366 = local write "log2-2"(w338) -> ()
                          }
                          frame #1 {
                            n367 = Greater?(x=w341, y=w340) -> (0:w342:bool)
                            n368 = case shown="True" w342 {
                              frame False {
                              }
                              frame True {
                                n369 = local write "LOG LAB02-2"("") -> ()
                                n370 = local write "log2-2"(0) -> ()
                              }
                            }
                          }
                        }
                      }
                      frame #1 {
                        w356 = "LAB02-2"
                        w348 = "/"
                        n371 = local read "DISP LAB02-2"() -> (w366:T4)
                        n372 = local read "SET LAB02-2"() -> (w360:T5)
                        n373 = Get Date/Time In Seconds() -> (seconds since 1Jan1904=w362:timestamp)
                        n374 = local write "LF2-2"(FALSE) -> ()
                        n375 = Unbundle(w360) -> ("NAME"=w347:string, "DESCRIPTION"=w346:string)  [unwired: 3 out]
                        n376 = Unbundle(w366) -> ("CYCLE"=w365:dbl, "MINS"=w364:dbl, "STATUS"=w351:string)
                        n377 = Get Date/Time String(seconds (now)=w362) -> (date string=w355:string, time string=w354:string)  [unwired: 2 in]
                        n378 = local read "LOG LAB02-2"() -> (w359:string)
                        n379 = Concatenate Strings(w347, w348, w346) -> (w345:string)
                        n380 = Number To Fractional String(number=w364, precision (6)=2) -> (F-format string=w352:string)  [unwired: 2 in]
                        n381 = Number To Decimal String(number=w365) -> (decimal integer string=w353:string)  [unwired: 1 in]
                        n382 = Bundle(w356, "date string"=w355, "time string"=w354, w345, w353, w352, "STATUS"=w351) -> (w350:T7)  [unwired: 1 in]
                        n383 = Concatenate Strings(w356, w348, w355, w348, w354, w348, w345, w348, w353, w348, w352, w348, w351, "\r\n") -> (w357:string)
                        n384 = Concatenate Strings(w359, w357) -> (w358:string)
                        n385 = local write "LOG LAB02-2"(w358) -> ()
                        n386 = call "sub vi - Log udate V2.vi"("data"=w350, "panel id"=w356) -> ("error out"=w349:errorcluster)  [unwired: 9 in]
                        n387 = local write "error out"(w349) -> ()
                      }
                    }
                  }
                }
                n388 = case shown="True" w331 {
                  frame False {
                  }
                  frame True {
                    n389 = local write "LF2-2"(TRUE) -> ()
                  }
                }
              }
              frame #4 {
                n390 = local read "RUN LAB03-1"() -> (w370:bool)
                n391 = local read "LF3-1"() -> (w372:bool)
                n392 = Not(x=w370) -> (.not. x?=w373:bool)
                n393 = And(x=w373, y=w372) -> (x .and. y?=w371:bool)
                n394 = case shown="True" w371 {
                  tunnel: w369 -> [_ w374]
                  frame False {
                  }
                  frame True {
                    n395 = stacked-sequence {
                      tunnel: w374 -> [w375 _]
                      frame #0 {
                        n396 = flat-sequence {
                          tunnel: [w377] -> w376
                          tunnel: w376 -> [w380]
                          tunnel: w375 -> [w379]
                          frame #0 {
                            n397 = local read "log3-1"() -> (w378:dbl)
                            n398 = Increment(x=w378) -> (x+1=w377:dbl)
                            n399 = local write "log3-1"(w377) -> ()
                          }
                          frame #1 {
                            n400 = Greater?(x=w380, y=w379) -> (0:w381:bool)
                            n401 = case shown="True" w381 {
                              frame False {
                              }
                              frame True {
                                n402 = local write "LOG LAB03-1"("") -> ()
                                n403 = local write "log3-1"(0) -> ()
                              }
                            }
                          }
                        }
                      }
                      frame #1 {
                        w395 = "LAB03-1"
                        w387 = "/"
                        n404 = local read "DISP LAB03-1"() -> (w405:T4)
                        n405 = local read "SET LAB03-1"() -> (w399:T5)
                        n406 = Get Date/Time In Seconds() -> (seconds since 1Jan1904=w401:timestamp)
                        n407 = local write "LF3-1"(FALSE) -> ()
                        n408 = Unbundle(w399) -> ("NAME"=w386:string, "DESCRIPTION"=w385:string)  [unwired: 3 out]
                        n409 = Unbundle(w405) -> ("CYCLE"=w404:dbl, "MINS"=w403:dbl, "STATUS"=w390:string)
                        n410 = Get Date/Time String(seconds (now)=w401) -> (date string=w394:string, time string=w393:string)  [unwired: 2 in]
                        n411 = local read "LOG LAB03-1"() -> (w398:string)
                        n412 = Concatenate Strings(w386, w387, w385) -> (w384:string)
                        n413 = Number To Fractional String(number=w403, precision (6)=2) -> (F-format string=w391:string)  [unwired: 2 in]
                        n414 = Number To Decimal String(number=w404) -> (decimal integer string=w392:string)  [unwired: 1 in]
                        n415 = Bundle(w395, "date string"=w394, "time string"=w393, w384, w392, w391, "STATUS"=w390) -> (w389:T7)  [unwired: 1 in]
                        n416 = Concatenate Strings(w395, w387, w394, w387, w393, w387, w384, w387, w392, w387, w391, w387, w390, "\r\n") -> (w396:string)
                        n417 = Concatenate Strings(w398, w396) -> (w397:string)
                        n418 = local write "LOG LAB03-1"(w397) -> ()
                        n419 = call "sub vi - Log udate V2.vi"("data"=w389, "panel id"=w395) -> ("error out"=w388:errorcluster)  [unwired: 9 in]
                        n420 = local write "error out"(w388) -> ()
                      }
                    }
                  }
                }
                n421 = case shown="True" w370 {
                  frame False {
                  }
                  frame True {
                    n422 = local write "LF3-1"(TRUE) -> ()
                  }
                }
              }
              frame #5 {
                n423 = local read "RUN LAB03-2"() -> (w409:bool)
                n424 = local read "LF3-2"() -> (w411:bool)
                n425 = Not(x=w409) -> (.not. x?=w412:bool)
                n426 = And(x=w412, y=w411) -> (x .and. y?=w410:bool)
                n427 = case shown="True" w410 {
                  tunnel: w408 -> [_ w413]
                  frame False {
                  }
                  frame True {
                    n428 = stacked-sequence {
                      tunnel: w413 -> [w414 _]
                      frame #0 {
                        n429 = flat-sequence {
                          tunnel: [w416] -> w415
                          tunnel: w415 -> [w419]
                          tunnel: w414 -> [w418]
                          frame #0 {
                            n430 = local read "log3-2"() -> (w417:dbl)
                            n431 = Increment(x=w417) -> (x+1=w416:dbl)
                            n432 = local write "log3-2"(w416) -> ()
                          }
                          frame #1 {
                            n433 = Greater?(x=w419, y=w418) -> (0:w420:bool)
                            n434 = case shown="True" w420 {
                              frame False {
                              }
                              frame True {
                                n435 = local write "LOG LAB03-2"("") -> ()
                                n436 = local write "log3-2"(0) -> ()
                              }
                            }
                          }
                        }
                      }
                      frame #1 {
                        w434 = "LAB03-2"
                        w426 = "/"
                        n437 = local read "DISP LAB03-2"() -> (w444:T4)
                        n438 = local read "SET LAB03-2"() -> (w438:T5)
                        n439 = Get Date/Time In Seconds() -> (seconds since 1Jan1904=w440:timestamp)
                        n440 = local write "LF3-2"(FALSE) -> ()
                        n441 = Unbundle(w438) -> ("NAME"=w425:string, "DESCRIPTION"=w424:string)  [unwired: 3 out]
                        n442 = Unbundle(w444) -> ("CYCLE"=w443:dbl, "MINS"=w442:dbl, "STATUS"=w429:string)
                        n443 = Get Date/Time String(seconds (now)=w440) -> (date string=w433:string, time string=w432:string)  [unwired: 2 in]
                        n444 = local read "LOG LAB03-2"() -> (w437:string)
                        n445 = Concatenate Strings(w425, w426, w424) -> (w423:string)
                        n446 = Number To Fractional String(number=w442, precision (6)=2) -> (F-format string=w430:string)  [unwired: 2 in]
                        n447 = Number To Decimal String(number=w443) -> (decimal integer string=w431:string)  [unwired: 1 in]
                        n448 = Bundle(w434, "date string"=w433, "time string"=w432, w423, w431, w430, "STATUS"=w429) -> (w428:T7)  [unwired: 1 in]
                        n449 = Concatenate Strings(w434, w426, w433, w426, w432, w426, w423, w426, w431, w426, w430, w426, w429, "\r\n") -> (w435:string)
                        n450 = Concatenate Strings(w437, w435) -> (w436:string)
                        n451 = local write "LOG LAB03-2"(w436) -> ()
                        n452 = call "sub vi - Log udate V2.vi"("data"=w428, "panel id"=w434) -> ("error out"=w427:errorcluster)  [unwired: 9 in]
                        n453 = local write "error out"(w427) -> ()
                      }
                    }
                  }
                }
                n454 = case shown="True" w409 {
                  frame False {
                  }
                  frame True {
                    n455 = local write "LF3-2"(TRUE) -> ()
                  }
                }
              }
              frame #6 {
                n456 = local read "RUN LAB04-1"() -> (w448:bool)
                n457 = local read "LF4-1"() -> (w450:bool)
                n458 = Not(x=w448) -> (.not. x?=w451:bool)
                n459 = And(x=w451, y=w450) -> (x .and. y?=w449:bool)
                n460 = case shown="True" w449 {
                  tunnel: w447 -> [_ w452]
                  frame False {
                  }
                  frame True {
                    n461 = stacked-sequence {
                      tunnel: w452 -> [w453 _]
                      frame #0 {
                        n462 = flat-sequence {
                          tunnel: [w455] -> w454
                          tunnel: w454 -> [w458]
                          tunnel: w453 -> [w457]
                          frame #0 {
                            n463 = local read "log4-1"() -> (w456:dbl)
                            n464 = Increment(x=w456) -> (x+1=w455:dbl)
                            n465 = local write "log4-1"(w455) -> ()
                          }
                          frame #1 {
                            n466 = Greater?(x=w458, y=w457) -> (0:w459:bool)
                            n467 = case shown="True" w459 {
                              frame False {
                              }
                              frame True {
                                n468 = local write "LOG LAB04-1"("") -> ()
                                n469 = local write "log4-1"(0) -> ()
                              }
                            }
                          }
                        }
                      }
                      frame #1 {
                        w473 = "LAB04-1"
                        w465 = "/"
                        n470 = local read "DISP LAB04-1"() -> (w483:T4)
                        n471 = local read "SET LAB04-1"() -> (w477:T5)
                        n472 = Get Date/Time In Seconds() -> (seconds since 1Jan1904=w479:timestamp)
                        n473 = local write "LF4-1"(FALSE) -> ()
                        n474 = Unbundle(w477) -> ("NAME"=w464:string, "DESCRIPTION"=w463:string)  [unwired: 3 out]
                        n475 = Unbundle(w483) -> ("CYCLE"=w482:dbl, "MINS"=w481:dbl, "STATUS"=w468:string)
                        n476 = Get Date/Time String(seconds (now)=w479) -> (date string=w472:string, time string=w471:string)  [unwired: 2 in]
                        n477 = local read "LOG LAB04-1"() -> (w476:string)
                        n478 = Concatenate Strings(w464, w465, w463) -> (w462:string)
                        n479 = Number To Fractional String(number=w481, precision (6)=2) -> (F-format string=w469:string)  [unwired: 2 in]
                        n480 = Number To Decimal String(number=w482) -> (decimal integer string=w470:string)  [unwired: 1 in]
                        n481 = Bundle(w473, "date string"=w472, "time string"=w471, w462, w470, w469, "STATUS"=w468) -> (w467:T7)  [unwired: 1 in]
                        n482 = Concatenate Strings(w473, w465, w472, w465, w471, w465, w462, w465, w470, w465, w469, w465, w468, "\r\n") -> (w474:string)
                        n483 = Concatenate Strings(w476, w474) -> (w475:string)
                        n484 = local write "LOG LAB04-1"(w475) -> ()
                        n485 = call "sub vi - Log udate V2.vi"("data"=w467, "panel id"=w473) -> ("error out"=w466:errorcluster)  [unwired: 9 in]
                        n486 = local write "error out"(w466) -> ()
                      }
                    }
                  }
                }
                n487 = case shown="True" w448 {
                  frame False {
                  }
                  frame True {
                    n488 = local write "LF4-1"(TRUE) -> ()
                  }
                }
              }
              frame #7 {
                n489 = local read "RUN LAB04-2"() -> (w487:bool)
                n490 = local read "LF4-2"() -> (w489:bool)
                n491 = Not(x=w487) -> (.not. x?=w490:bool)
                n492 = And(x=w490, y=w489) -> (x .and. y?=w488:bool)
                n493 = case shown="True" w488 {
                  tunnel: w486 -> [_ w491]
                  frame False {
                  }
                  frame True {
                    n494 = stacked-sequence {
                      tunnel: w491 -> [w492 _]
                      frame #0 {
                        n495 = flat-sequence {
                          tunnel: [w494] -> w493
                          tunnel: w493 -> [w497]
                          tunnel: w492 -> [w496]
                          frame #0 {
                            n496 = local read "log4-2"() -> (w495:dbl)
                            n497 = Increment(x=w495) -> (x+1=w494:dbl)
                            n498 = local write "log4-2"(w494) -> ()
                          }
                          frame #1 {
                            n499 = Greater?(x=w497, y=w496) -> (0:w498:bool)
                            n500 = case shown="True" w498 {
                              frame False {
                              }
                              frame True {
                                n501 = local write "LOG LAB04-2"("") -> ()
                                n502 = local write "log4-2"(0) -> ()
                              }
                            }
                          }
                        }
                      }
                      frame #1 {
                        w512 = "LAB04-2"
                        w504 = "/"
                        n503 = local read "DISP LAB04-2"() -> (w522:T4)
                        n504 = local read "SET LAB04-2"() -> (w516:T5)
                        n505 = Get Date/Time In Seconds() -> (seconds since 1Jan1904=w518:timestamp)
                        n506 = local write "LF4-2"(FALSE) -> ()
                        n507 = Unbundle(w516) -> ("NAME"=w503:string, "DESCRIPTION"=w502:string)  [unwired: 3 out]
                        n508 = Unbundle(w522) -> ("CYCLE"=w521:dbl, "MINS"=w520:dbl, "STATUS"=w507:string)
                        n509 = Get Date/Time String(seconds (now)=w518) -> (date string=w511:string, time string=w510:string)  [unwired: 2 in]
                        n510 = local read "LOG LAB04-2"() -> (w515:string)
                        n511 = Concatenate Strings(w503, w504, w502) -> (w501:string)
                        n512 = Number To Fractional String(number=w520, precision (6)=2) -> (F-format string=w508:string)  [unwired: 2 in]
                        n513 = Number To Decimal String(number=w521) -> (decimal integer string=w509:string)  [unwired: 1 in]
                        n514 = Bundle(w512, "date string"=w511, "time string"=w510, w501, w509, w508, "STATUS"=w507) -> (w506:T7)  [unwired: 1 in]
                        n515 = Concatenate Strings(w512, w504, w511, w504, w510, w504, w501, w504, w509, w504, w508, w504, w507, "\r\n") -> (w513:string)
                        n516 = Concatenate Strings(w515, w513) -> (w514:string)
                        n517 = local write "LOG LAB04-2"(w514) -> ()
                        n518 = call "sub vi - Log udate V2.vi"("data"=w506, "panel id"=w512) -> ("error out"=w505:errorcluster)  [unwired: 9 in]
                        n519 = local write "error out"(w505) -> ()
                      }
                    }
                  }
                }
                n520 = case shown="True" w487 {
                  frame False {
                  }
                  frame True {
                    n521 = local write "LF4-2"(TRUE) -> ()
                  }
                }
              }
              frame #8 {
                n522 = local read "RUN LAB05-1"() -> (w526:bool)
                n523 = local read "LF5-1"() -> (w528:bool)
                n524 = Not(x=w526) -> (.not. x?=w529:bool)
                n525 = And(x=w529, y=w528) -> (x .and. y?=w527:bool)
                n526 = case shown="True" w527 {
                  tunnel: w525 -> [_ w530]
                  frame False {
                  }
                  frame True {
                    n527 = stacked-sequence {
                      tunnel: w530 -> [w531 _]
                      frame #0 {
                        n528 = flat-sequence {
                          tunnel: [w533] -> w532
                          tunnel: w532 -> [w536]
                          tunnel: w531 -> [w535]
                          frame #0 {
                            n529 = local read "log5-1"() -> (w534:dbl)
                            n530 = Increment(x=w534) -> (x+1=w533:dbl)
                            n531 = local write "log5-1"(w533) -> ()
                          }
                          frame #1 {
                            n532 = Greater?(x=w536, y=w535) -> (0:w537:bool)
                            n533 = case shown="True" w537 {
                              frame False {
                              }
                              frame True {
                                n534 = local write "LOG LAB05-1"("") -> ()
                                n535 = local write "log5-1"(0) -> ()
                              }
                            }
                          }
                        }
                      }
                      frame #1 {
                        w551 = "LAB05-1"
                        w543 = "/"
                        n536 = local read "DISP LAB05-1"() -> (w561:T4)
                        n537 = local read "SET LAB05-1"() -> (w555:T5)
                        n538 = Get Date/Time In Seconds() -> (seconds since 1Jan1904=w557:timestamp)
                        n539 = local write "LF5-1"(FALSE) -> ()
                        n540 = Unbundle(w555) -> ("NAME"=w542:string, "DESCRIPTION"=w541:string)  [unwired: 3 out]
                        n541 = Unbundle(w561) -> ("CYCLE"=w560:dbl, "MINS"=w559:dbl, "STATUS"=w546:string)
                        n542 = Get Date/Time String(seconds (now)=w557) -> (date string=w550:string, time string=w549:string)  [unwired: 2 in]
                        n543 = local read "LOG LAB05-1"() -> (w554:string)
                        n544 = Concatenate Strings(w542, w543, w541) -> (w540:string)
                        n545 = Number To Fractional String(number=w559, precision (6)=2) -> (F-format string=w547:string)  [unwired: 2 in]
                        n546 = Number To Decimal String(number=w560) -> (decimal integer string=w548:string)  [unwired: 1 in]
                        n547 = Bundle(w551, "date string"=w550, "time string"=w549, w540, w548, w547, "STATUS"=w546) -> (w545:T7)  [unwired: 1 in]
                        n548 = Concatenate Strings(w551, w543, w550, w543, w549, w543, w540, w543, w548, w543, w547, w543, w546, "\r\n") -> (w552:string)
                        n549 = Concatenate Strings(w554, w552) -> (w553:string)
                        n550 = local write "LOG LAB05-1"(w553) -> ()
                        n551 = call "sub vi - Log udate V2.vi"("data"=w545, "panel id"=w551) -> ("error out"=w544:errorcluster)  [unwired: 9 in]
                        n552 = local write "error out"(w544) -> ()
                      }
                    }
                  }
                }
                n553 = case shown="True" w526 {
                  frame False {
                  }
                  frame True {
                    n554 = local write "LF5-1"(TRUE) -> ()
                  }
                }
              }
              frame #9 {
                n555 = local read "RUN LAB05-2"() -> (w565:bool)
                n556 = local read "LF5-2"() -> (w567:bool)
                n557 = Not(x=w565) -> (.not. x?=w568:bool)
                n558 = And(x=w568, y=w567) -> (x .and. y?=w566:bool)
                n559 = case shown="True" w566 {
                  tunnel: w564 -> [_ w569]
                  frame False {
                  }
                  frame True {
                    n560 = stacked-sequence {
                      tunnel: w569 -> [w570 _]
                      frame #0 {
                        n561 = flat-sequence {
                          tunnel: [w572] -> w571
                          tunnel: w571 -> [w575]
                          tunnel: w570 -> [w574]
                          frame #0 {
                            n562 = local read "log5-2"() -> (w573:dbl)
                            n563 = Increment(x=w573) -> (x+1=w572:dbl)
                            n564 = local write "log5-2"(w572) -> ()
                          }
                          frame #1 {
                            n565 = Greater?(x=w575, y=w574) -> (0:w576:bool)
                            n566 = case shown="True" w576 {
                              frame False {
                              }
                              frame True {
                                n567 = local write "LOG LAB05-2"("") -> ()
                                n568 = local write "log5-2"(0) -> ()
                              }
                            }
                          }
                        }
                      }
                      frame #1 {
                        w590 = "LAB05-2"
                        w582 = "/"
                        n569 = local read "DISP LAB05-2"() -> (w600:T4)
                        n570 = local read "SET LAB05-2"() -> (w594:T5)
                        n571 = Get Date/Time In Seconds() -> (seconds since 1Jan1904=w596:timestamp)
                        n572 = local write "LF5-2"(FALSE) -> ()
                        n573 = Unbundle(w594) -> ("NAME"=w581:string, "DESCRIPTION"=w580:string)  [unwired: 3 out]
                        n574 = Unbundle(w600) -> ("CYCLE"=w599:dbl, "MINS"=w598:dbl, "STATUS"=w585:string)
                        n575 = Get Date/Time String(seconds (now)=w596) -> (date string=w589:string, time string=w588:string)  [unwired: 2 in]
                        n576 = local read "LOG LAB05-2"() -> (w593:string)
                        n577 = Concatenate Strings(w581, w582, w580) -> (w579:string)
                        n578 = Number To Fractional String(number=w598, precision (6)=2) -> (F-format string=w586:string)  [unwired: 2 in]
                        n579 = Number To Decimal String(number=w599) -> (decimal integer string=w587:string)  [unwired: 1 in]
                        n580 = Bundle(w590, "date string"=w589, "time string"=w588, w579, w587, w586, "STATUS"=w585) -> (w584:T7)  [unwired: 1 in]
                        n581 = Concatenate Strings(w590, w582, w589, w582, w588, w582, w579, w582, w587, w582, w586, w582, w585, "\r\n") -> (w591:string)
                        n582 = Concatenate Strings(w593, w591) -> (w592:string)
                        n583 = local write "LOG LAB05-2"(w592) -> ()
                        n584 = call "sub vi - Log udate V2.vi"("data"=w584, "panel id"=w590) -> ("error out"=w583:errorcluster)  [unwired: 9 in]
                        n585 = local write "error out"(w583) -> ()
                      }
                    }
                  }
                }
                n586 = case shown="True" w565 {
                  frame False {
                  }
                  frame True {
                    n587 = local write "LF5-2"(TRUE) -> ()
                  }
                }
              }
            }
          }
          frame #3 {
            # "save current log files to network dir for viewing"
            # "save last months log files to networ dir for new month"
            # "send log data to main program"
            n588 = local read "LOG LAB05-2"() -> (w617:string)
            n589 = local read "LOG LAB02-1"() -> (w624:string)
            n590 = local read "LOG LAB03-2"() -> (w621:string)
            n591 = local read "LOG LAB04-1"() -> (w620:string)
            n592 = local read "LOG LAB05-1"() -> (w618:string)
            n593 = local read "LOG LAB02-2"() -> (w623:string)
            n594 = local read "LOG LAB04-2"() -> (w619:string)
            n595 = local read "LOG LAB03-1"() -> (w622:string)
            n596 = local read "LOG LAB01-2"() -> (w625:string)
            n597 = local read "LOG LAB01-1"() -> (w626:string)
            n598 = global write "Global display 3.vi" "log 5-2"(w617) -> ()
            n599 = global write "Global display 3.vi" "log 4-2"(w619) -> ()
            n600 = global write "Global display 3.vi" "log 1-1"(w626) -> ()
            n601 = global write "Global display 3.vi" "log 5-1"(w618) -> ()
            n602 = global write "Global display 3.vi" "log 1-2"(w625) -> ()
            n603 = global write "Global display 3.vi" "log 4-1"(w620) -> ()
            n604 = global write "Global display 3.vi" "log 2-2"(w623) -> ()
            n605 = global write "Global display 3.vi" "log 2-1"(w624) -> ()
            n606 = global write "Global display 3.vi" "log 3-1"(w622) -> ()
            n607 = global write "Global display 3.vi" "log 3-2"(w621) -> ()
            n608 = property on="Tab Control 2" class="TabCtl (strict)"() -> ("Pages"=w606:refnum<vi>[])  [unwired: 2 in, 2 out]
            n609 = global read "Global display 3.vi" "admin"() -> (w603:bool)
            n610 = Index Array(array=w606, index=9) -> (element=w604:refnum<vi>)
            n611 = property class="Page"(reference=w604, "PageVis"=w603) -> ()  [unwired: 1 in, 2 out]
            n612 = Get Date/Time In Seconds() -> (seconds since 1Jan1904=w614:timestamp)
            n613 = case shown="True" "Save Log File\nTo Disk For\nViewing" {
              frame False {
              }
              frame True {
                n614 = stacked-sequence {
                  seq-local: [w632 _] -> [_ w635]
                  frame #0 {
                    n615 = call "sub vi - save log files V1.vi"() -> ("error out"=w631:errorcluster, "network dir"=w632:string)  [unwired: 9 in]
                    n616 = call <vilib>:"Simple Error Handler.vi"("error in (no error)"=w631) -> ()  [unwired: 4 in, 5 out]
                  }
                  frame #1 {
                    n617 = local write "Save Log File\nTo Disk For\nViewing"(FALSE) -> ()
                    n618 = Concatenate Strings("Saved:", w635) -> (w634:string)
                    n619 = One Button Dialog(message=w634) -> ()  [unwired: 1 in, 1 out]
                  }
                }
              }
            }
            n620 = Format Date/Time String(time format string (%c)="\\LabPanel%Y\\%b", seconds (now)=w614) -> (date/time string=w607:string)  [unwired: 1 in]
            n621 = local read "log file dir"() -> (w611:string)
            n622 = Equal?(x=w611, y="") -> (x = y?=w612:bool)
            n623 = Select(t=w607, s=w612, f=w611) -> (s? t:f=→"log file dir":string)
            n624 = local read "log file dir"() -> (w608:string)
            n625 = Not Equal?(x=w607, y=w608) -> (x != y?=w609:bool)
            n626 = case shown="True" w609 {
              tunnel: w608 -> [_ w628]
              tunnel: w607 -> [_ w627]
              frame False {
              }
              frame True {
                n627 = stacked-sequence {
                  tunnel: w628 -> [w629 _]
                  tunnel: w627 -> [_ w630]
                  frame #0 {
                    n628 = call "sub vi - save log dir V1.vi"("Dir Input"=w629) -> ()  [unwired: 11 in]
                  }
                  frame #1 {
                    n629 = local write "log file dir"(w630) -> ()
                  }
                }
              }
            }
          }
        }
        n630 = global read "Global display 1.vi" "stop disp"() -> (w2:bool)
        n631 = Or(x="Stop Button", y=w2) -> (x .or. y?=w4:bool)
      }
    }
  }
